vi "Main_UCRT_9.vi"() -> ()   [LabVIEW 2016]
doc: "Use this template to create an application that executes until you click the Stop button. Unlike the Single Loop Application VI that uses polling, this VI uses the Event Structure."
uses:
  <vilib>/vision/driver/NI_Vision_Acquisition_Software.lvlib
  <vilib>/vision/NI_Vision_Development_Module.lvlib
  Granule-2000AT/PC/Library.lvlib
  <vilib>/Utility/file.llb/Write To Spreadsheet File (string).vi
  <vilib>/Utility/file.llb/Read From Spreadsheet File (string).vi
  <vilib>/userdefined/High Color/IMAQdx.ctl
panel:
  in  "ND HEAT BUT":bool
  in  "ND HEAT LED":bool
  out "PT 4txt":string caption="Вакуум в камере\nPT2 (torr)"
  out "PT4 2":u16(ring)
  out "NL2":u16(ring)
  in  "V5014":dbl
  out "давление 2":bool
  out "давление 1":bool
  in  "V5012_SP_He_PC2":dbl
  out "Air":bool
  in  "ПЛАЗМАТРОН В ИСХОДНОЕ":bool
  in  "Продол назад":bool
  in  "V5011_SP_He_PC2":dbl
  in  "V5010_SP_C1":dbl
  out "PT 4":string caption="Вакуум в камере\nPT2 (torr)"
  in  "PT4":dbl
  in  "M_PLasmatron":dbl
  out "V барабаны 2":dbl
  in  "Tab Control 2":enum32{"X1", "X2", "Y"}(tab)
  out "X240":bool[](array[boolean])
  out "ОП1 Х1 5":string[](array[string])
  out "X200":bool[](array[boolean])
  out "ОП1 Х1 4":string[](array[string])
  out "X140":bool[](array[boolean])
  out "ОП1 Х1 3":string[](array[string])
  out "X100":bool[](array[boolean])
  out "ОП1 Х1 2":string[](array[string])
  out "X400":bool[](array[boolean])
  out "ОП1 Х1 8":string[](array[string])
  out "X340":bool[](array[boolean])
  out "ОП1 Х1 7":string[](array[string])
  out "X300":bool[](array[boolean])
  out "ОП1 Х1 6":string[](array[string])
  out "Y120":bool[](array[boolean])
  out "ОП1 Х1 10":string[](array[string])
  out "Y60":bool[](array[boolean])
  out "ОП1 Х1 9":string[](array[string])
  out "Air 4":bool
  in  "PT3 2":dbl
  in  "Запись отчета":bool
  out "V вращ. бараб 2":string caption="V заготовки"
  out "LONGITUDINAL SPEED":string
  out "PLASMATRON SPEED":string
  in  "mac3":bool
  in  "Ошибка 2":i16 format="%x"
  in  "Скорость пп 2":i16
  out "Полож заг сер":bool
  out "Полож заг нач":bool caption="НАЧАЛО"
  out "Полож заг кон":bool
  out "Полож плазм кон":bool caption="Конец"
  out "Полож плазм сер":bool caption="Пром."
  out "Полож плазм  нач":bool caption="Начало"
  in  "МАКСИМАЛЬНАЯ СКОРОСТЬ ПП К":bool
  in  "v4066_cкорость подачи плазматрона":dbl
  in  "v4065_cкорость подачи":dbl
  in  "V7045_I_ist":dbl
  in  "V7045_U_ist":dbl
  in  "Действующий ток на плазматроне":string caption="Ток А"
  out "V заготовки":string
  in  "D, заготовки":i16
  in  "Закончить автораспыление":bool
  in  "Автораспыление доплавить":bool
  in  "Автораспыление начать":bool
  in  "задание тока А":string caption="Задание, А"
  in  "ПОДАЧА ЗАГОТОВКИ":bool
  in  "stop 3":bool
  in  "stop 2":bool
  in  "SP_зазор":dbl
  in  "PV_зазор":dbl
  in  "max out":dbl
  in  "out":dbl
  out "Distance зазор":sgl format="%.2f"
  out "x/y":dbl
  out "x*y":dbl
  out "16bit integer":i16
  in  "Numeric":i16
  in  "Т6":dbl
  in  "Улавливатель закрыть":bool
  in  "Улавливатель открыть":bool
  in  "Ролик прижать":bool
  in  "Ролик отжать":bool
  in  "PE3":dbl
  in  "PE2":dbl
  in  "PE1":dbl
  in  "ЗАДАНИЕ ТОКА":i16
  in  "ГС - Закрыть":bool
  in  "ГС -Открыть":bool
  out "ГС - Плазматрон":string caption="Плазматрон"
  out "ГС - Камера":string caption="Камера"
  in  "Скорость пп":i16
  in  "V барабаны задание":dbl
  in  "Выход":bool
  in  "ГС ПТ":i16
  in  "ГС камера":i16
  in  "V барабаны":dbl
  in  "Т5":dbl
  in  "Т4":dbl
  in  "Т3":dbl
  in  "Т2":dbl
  in  "Т1":dbl
  in  "Ошибка":i16
  in  "PT3":dbl
  in  "PT2":dbl
  in  "PT1":dbl
  in  "y120":i32
  in  "y60":i32
  in  "x400":i32
  in  "x340":i32
  in  "x300":i32
  in  "x240":i32
  in  "x200":i32
  in  "x140":i32
  in  "x100":i32
  in  "Tab Control":enum32{"Вакуум", "Распыление", "Осциллограмма"}(tab)
  in  "откачка стоп 2":bool
  out "Распыление":bool
  out "Вакуум":bool
  out "Газ":bool
  out "VP4":u16(ring)
  out "SP Presure Ar PC2":string caption="SP C1 (kgf/cm^2)"
  in  "напустить аргон в ресивер":bool
  in  "mac6":bool
  out "SP Presure He PC2":string caption="SP C1 (kgf/cm^2)"
  in  "mac5":bool
  in  "напустить гелий в ресивер":bool
  out "SP Presure C1":string caption="SP C1 (kgf/cm^2)"
  in  "mac 4":bool
  in  "напустить газ в камеру":bool
  out "PD2":u16(ring)
  out "VP2":u16(ring)
  in  "forvacuum":bool
  in  "forvakuum led":bool
  in  "Slide":dbl(slide) scale=0.0..99.0
  in  "откачка стоп":bool
  in  "откачка стоп индик":bool
  out "EV1":u16(ring)
  out "EV2":u16(ring)
  out "EV3.3":u16(ring)
  out "EV3.2":u16(ring)
  out "PE2":u16(ring)
  out "PE2":string caption="Вакуум в камере\nPT2 (torr)"
  out "CO1":u16(ring)
  out "CO2":u16(ring)
  out "EV3.1":u16(ring)
  out "CO3":u16(ring)
  out "P1":u16(ring)
  out "PE1":u16(ring)
  out "PE1":string caption="Вакуум в камере\nPT2 (torr)"
  out "PE3":u16(ring)
  out "PE3":string caption="Вакуум в камере\nPT2 (torr)"
  out "VP1":u16(ring)
  out "PT3":u16(ring)
  out "PT2":u16(ring)
  out "PT 2":string caption="Вакуум в камере\nPT2 (torr)"
  out "VP3":u16(ring)
  out "VP5":u16(ring)
  out "PD1":u16(ring)
  out "PT1":u16(ring)
  out "PT 1":string caption="Вакуум в камере\nPT2 (torr)"
  out "NZ1":u16(ring)
  out "NR1":u16(ring)
  out "NL1":u16(ring)
  in  "откачать рабочий вакуум":bool
  in  "mac 2":bool
  out "PT 3":string caption="Вакуум в камере\nPT2 (torr)"
  out "ИНдикатор положения полки":string
  in  "ЗУ-вверх":bool
  in  "Пауза допыления":string caption="Пауза допыления (sec)"
  out "C212":bool
  out "УГ_закрыт":bool caption="Отжат"
  out "УГ_открыт":bool caption="Прижат"
  out "ролик_отжат":bool caption="Вверху"
  out "ролик_прижат":bool caption="Внизу"
  out "max Speed":string caption="Максимальная \nСкорость (r/min)"
  out "ТЕМП КАМЕРА":string caption="T газ (C°)"
  in  "Скорость ПП 2":string caption="Скорость плазматрона\n(mm/min)"
  in  "Скорость ПП":string caption="Скорость толкателя (mm/min)"
  out "ТЕМП РОЛИК":string caption="T ролик (C°)"
  out "ПОДШ. 2.2":string caption="T4 (C°)"
  out "ПОДШ. 2.1":string caption="T3 (C°)"
  out "ПОДШ. 1.2":string caption="T2 (C°)"
  out "ПОДШ. 1.1":string caption="T1 (C°)"
  out "P плазматрон (bar)":string
  out "P камера (bar)":string
  out "I_ist":string caption="Ток (A)"
  out "U_ist":string caption="Напряжение (V)"
  in  "Tab Control 3":enum32{"Настройки видео", "Регулятор"}(tab)
  in  "Media Stop Button":bool
  in  "Play Button":bool
  in  "Камера":T1
  in  "Область измерения":T2 {"Rotation" format="%.2f"; "Left" scale=0.0..1024.0; "Right" scale=0.0..1280.0}
  in  "Параметры измерения":T3={"Contrast"=40, "Filter width"=4, "Steepness"=2, "Subsampling Ratio"=5, "Show Search Area"=FALSE, "Show Search Lines"=FALSE, "Show Edges Found"=FALSE, "Show Result"=TRUE}
  in  "Рабочий цвет":u32(colorbox)
  in  "Калибровка":u32(colorbox)
  in  "Задержка":u32
  in  "Уровень бинаризации":T4={"Нижний предел"=128.0, "Верхний предел"=255.0} {"Верхний предел" format="%.2f"; "Нижний предел" format="%.2f"}
  in  "Фильтр":i32(ring)=1 items=["Red", "Green", "Blue", "Hue", "Saturation", "Luminance", "Value", "Intensity"]
  out "Индикатор камеры":bool
  in  "Blank Button":bool
  out "Индикатор камеры 2":bool
  in  "Сохранить настройки":bool
  in  "автоматическое включение регулятора":bool caption="Автоматическое включение регулятора"
  out "Индикатор автозапуска регулятора":bool
  out "Запись":bool
  out "Максимальная подача (мм/мин)2":string caption="Max скорость\n(mm/min)"
  out "Boolean":bool
  in  "Регулятор":bool
  out "текущая скорость\n(mm/min)":string
  out "текущее значение\nзазора (mm)":string
  out "Задание \nзазора (mm)":string
  in  "взять зазор":bool caption="Регулятор"
  out "Марка сплава":string
  out "Порядковый номер":string caption="Номер цикла (un)"
  in  "Положение толкателя (mm)":dbl(slide) scale=0.0..100.0
  out "Диаметр заг.":string caption="Диаметр (mm)"
  out "V задания":string caption="Скорость вращения (r/min)"
  out "V вращ. бараб":string caption="Частота вращения (r/min)"
  in  "Продол впер":bool
  out "индикация видео":T5(plugin-control)
  in  "ПЛАЗМАТРОН В ИСХОДНОЕ 2":bool
  out "Частота вращения":dbl(graph)
  out "Значение зазора":dbl(graph)
  out "Скорость толкателя":dbl(graph)
  out "Ток":dbl(graph)
  out "Напряжение":dbl(graph)
  out "voto plasmatron":string caption="моточасы работы\nплазматрона"
  out "текущее время":string
  in  "Arhive":bool
  # "Ролик"
  # "Улавливатель ОГ"
  # "PLASMATRON"
  # "Обработка"
  # "БАРАБАНЫ"
  # "РАСПЫЛЕНИЕ ЗАГОТОВКИ"
  # "Температура"
  # "3A3.1 X100-X137"
  # "3A3.2 X140-177"
  # "3A4 X200-X237"
  # "3A5.1 X240-X277"
  # "3A5.2 X300-X337"
  # "3A6 X340-X377"
  # "3A8 X400-X437"
  # "2A8 Y60-Y117"
  # "3A7 Y120-Y157"
  # "Положение толкателя"
  # "Положение плазматрона"
  # "Газовая система"
  # "VF1"
  # "Ar,He"
  # "PC1"
  # "PC2"
  # "Толкатель"
  # "Прижим крышки"
  # "Прижимной ролик"
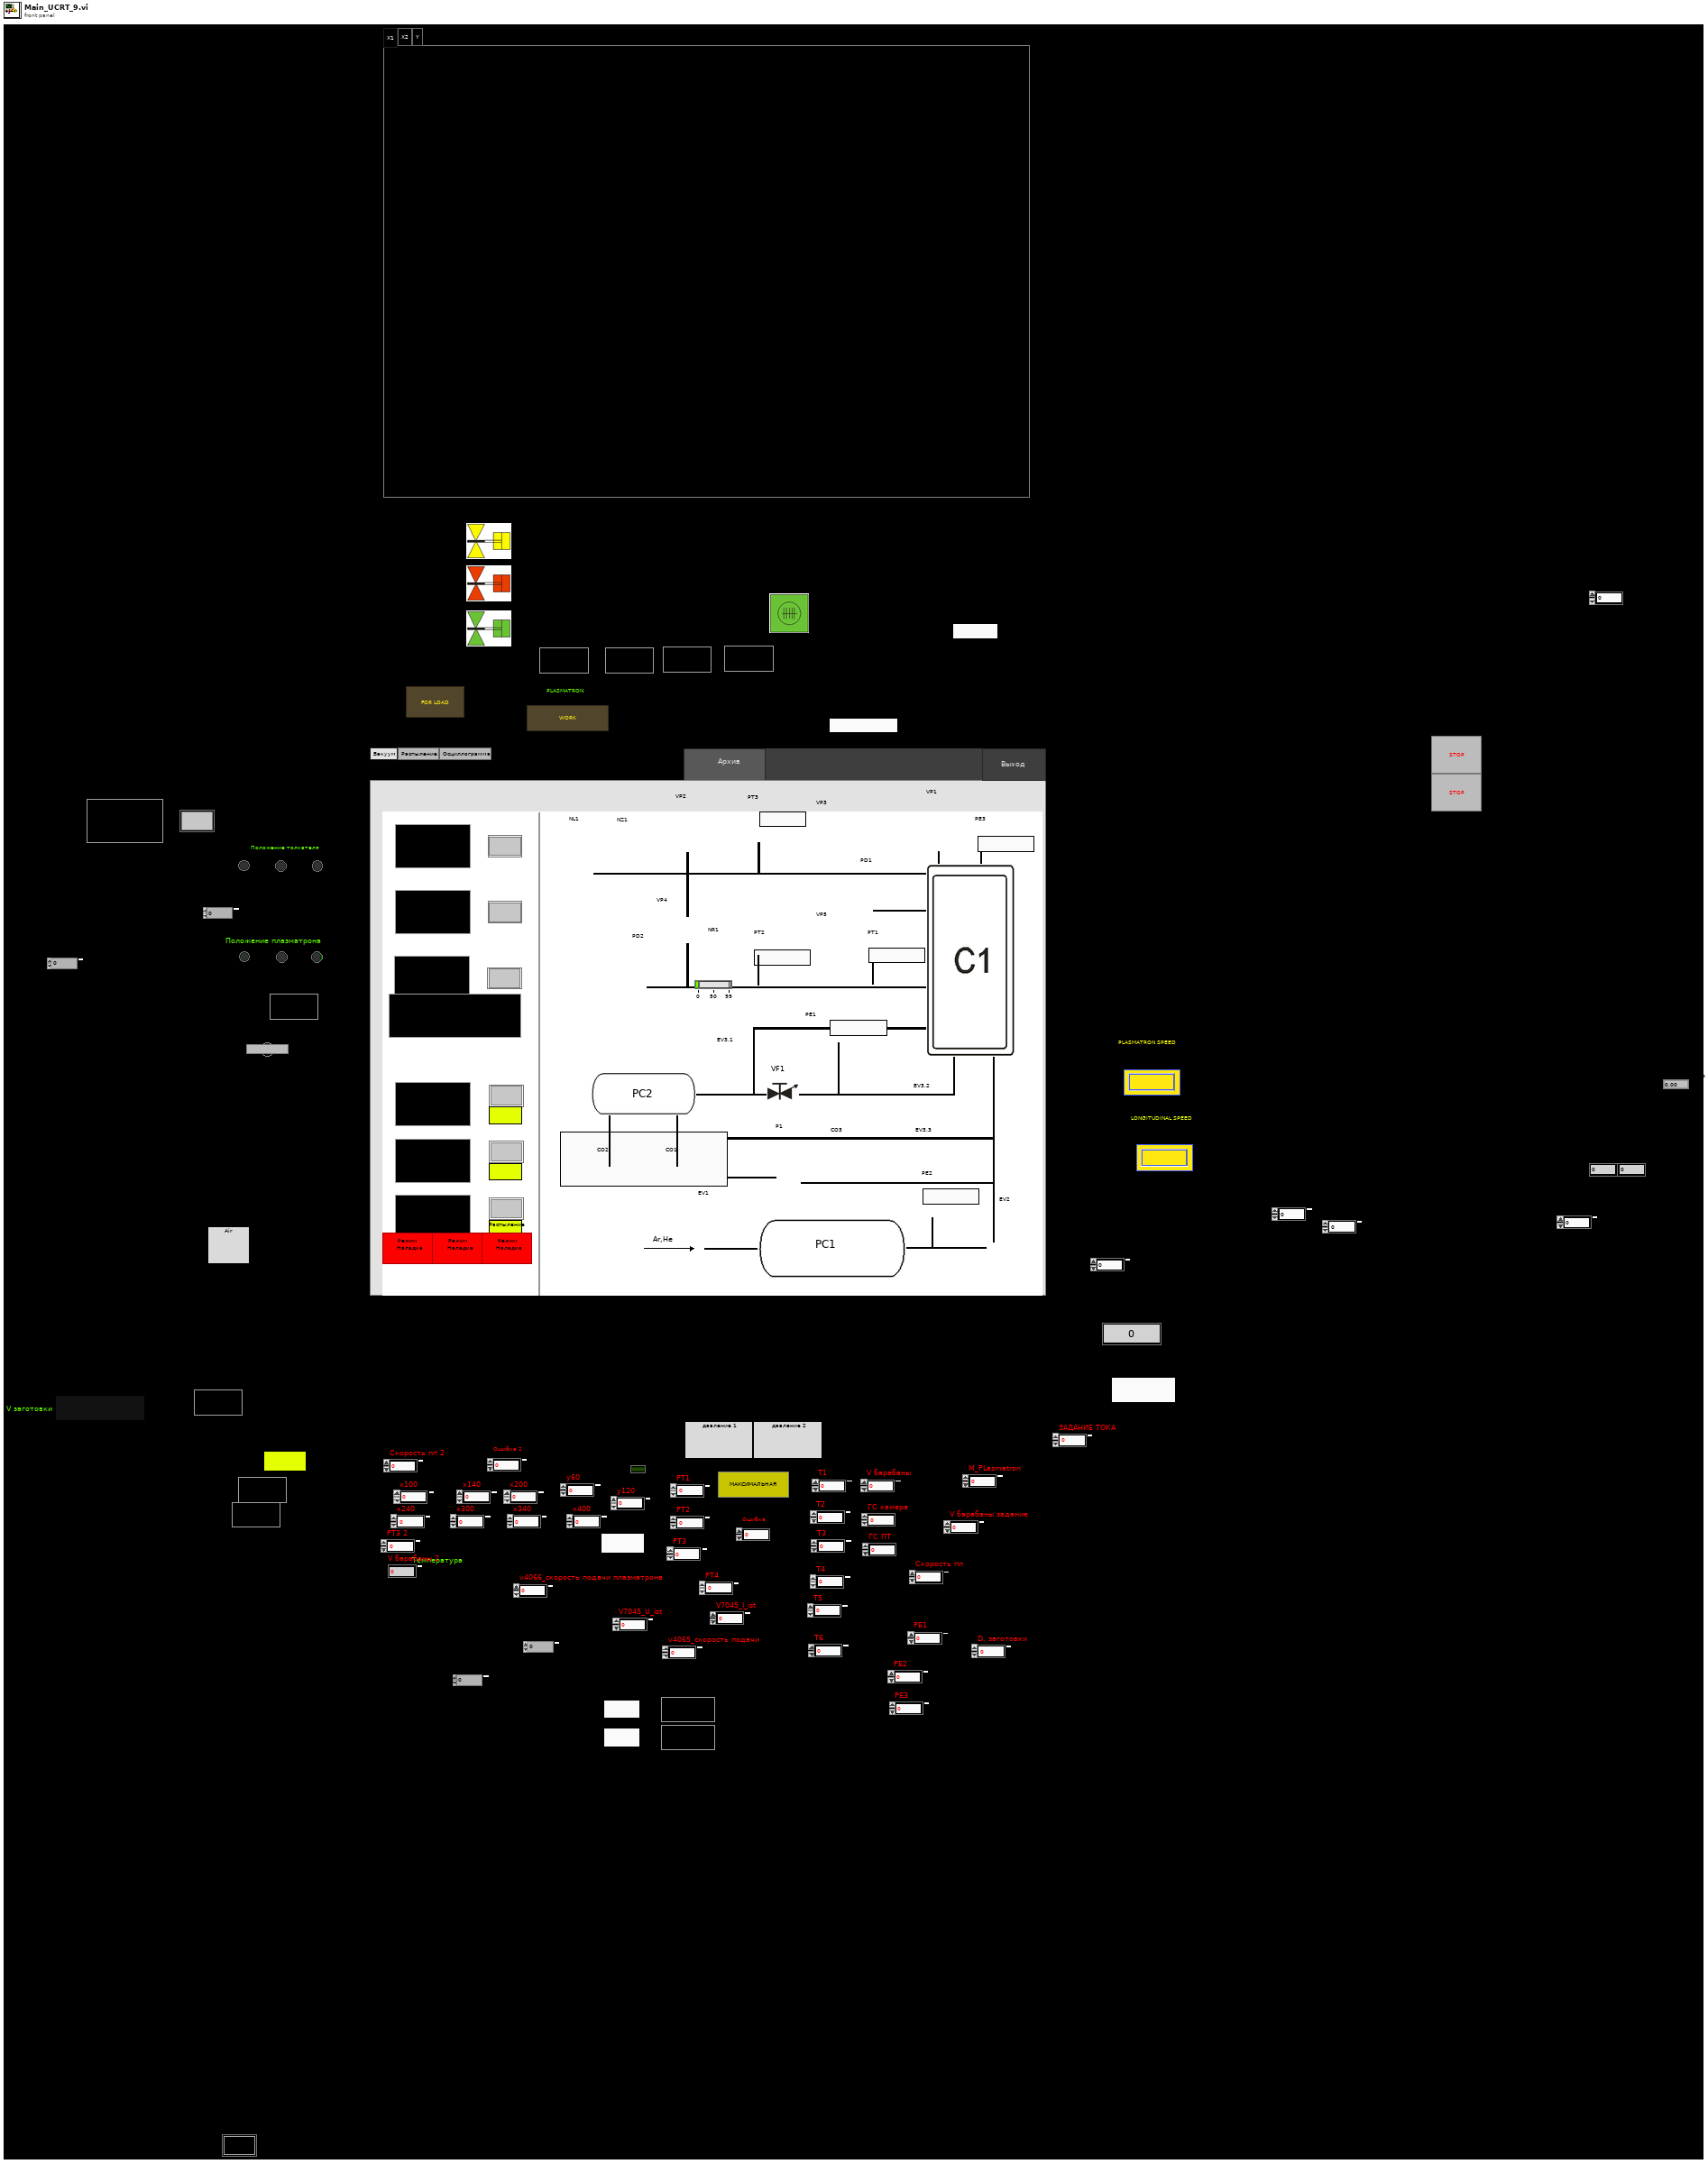
[diagram p1: front panel]
types:
  T1 = typedef "IMAQdx.ctl" = refnum<k21>
  T2 = typedef "IMAQ Rectangle" = cluster{"Left":i32, "Top":i32, "Right":i32, "Bottom":i32, "Rotation":dbl}
  T3 = cluster{"Contrast":i32, "Filter width":i32, "Steepness":i32, "Subsampling Ratio":u32, "Show Search Area":bool, "Show Search Lines":bool, "Show Edges Found":bool, "Show Result":bool}
  T4 = cluster{"Нижний предел":sgl, "Верхний предел":sgl}
  T5 = typedef "IMAQ Image.ctl" = refnum<image>
  T6 = enum16{"open", "replace", "create", "open or create", "replace or create", "replace or create with confirmation"}
  T7 = enum8{"Enabled", "Disabled", "Disabled and Grayed Out"}
  T8 = cluster{i32, i32, i32, u32, "Boolean":bool, "Boolean":bool, "Boolean":bool, "Boolean":bool}
  T9 = typedef "Image Type" = u32
  T10 = typedef "Library.lvlib/IMAQdx.ctl" = refnum<k21>
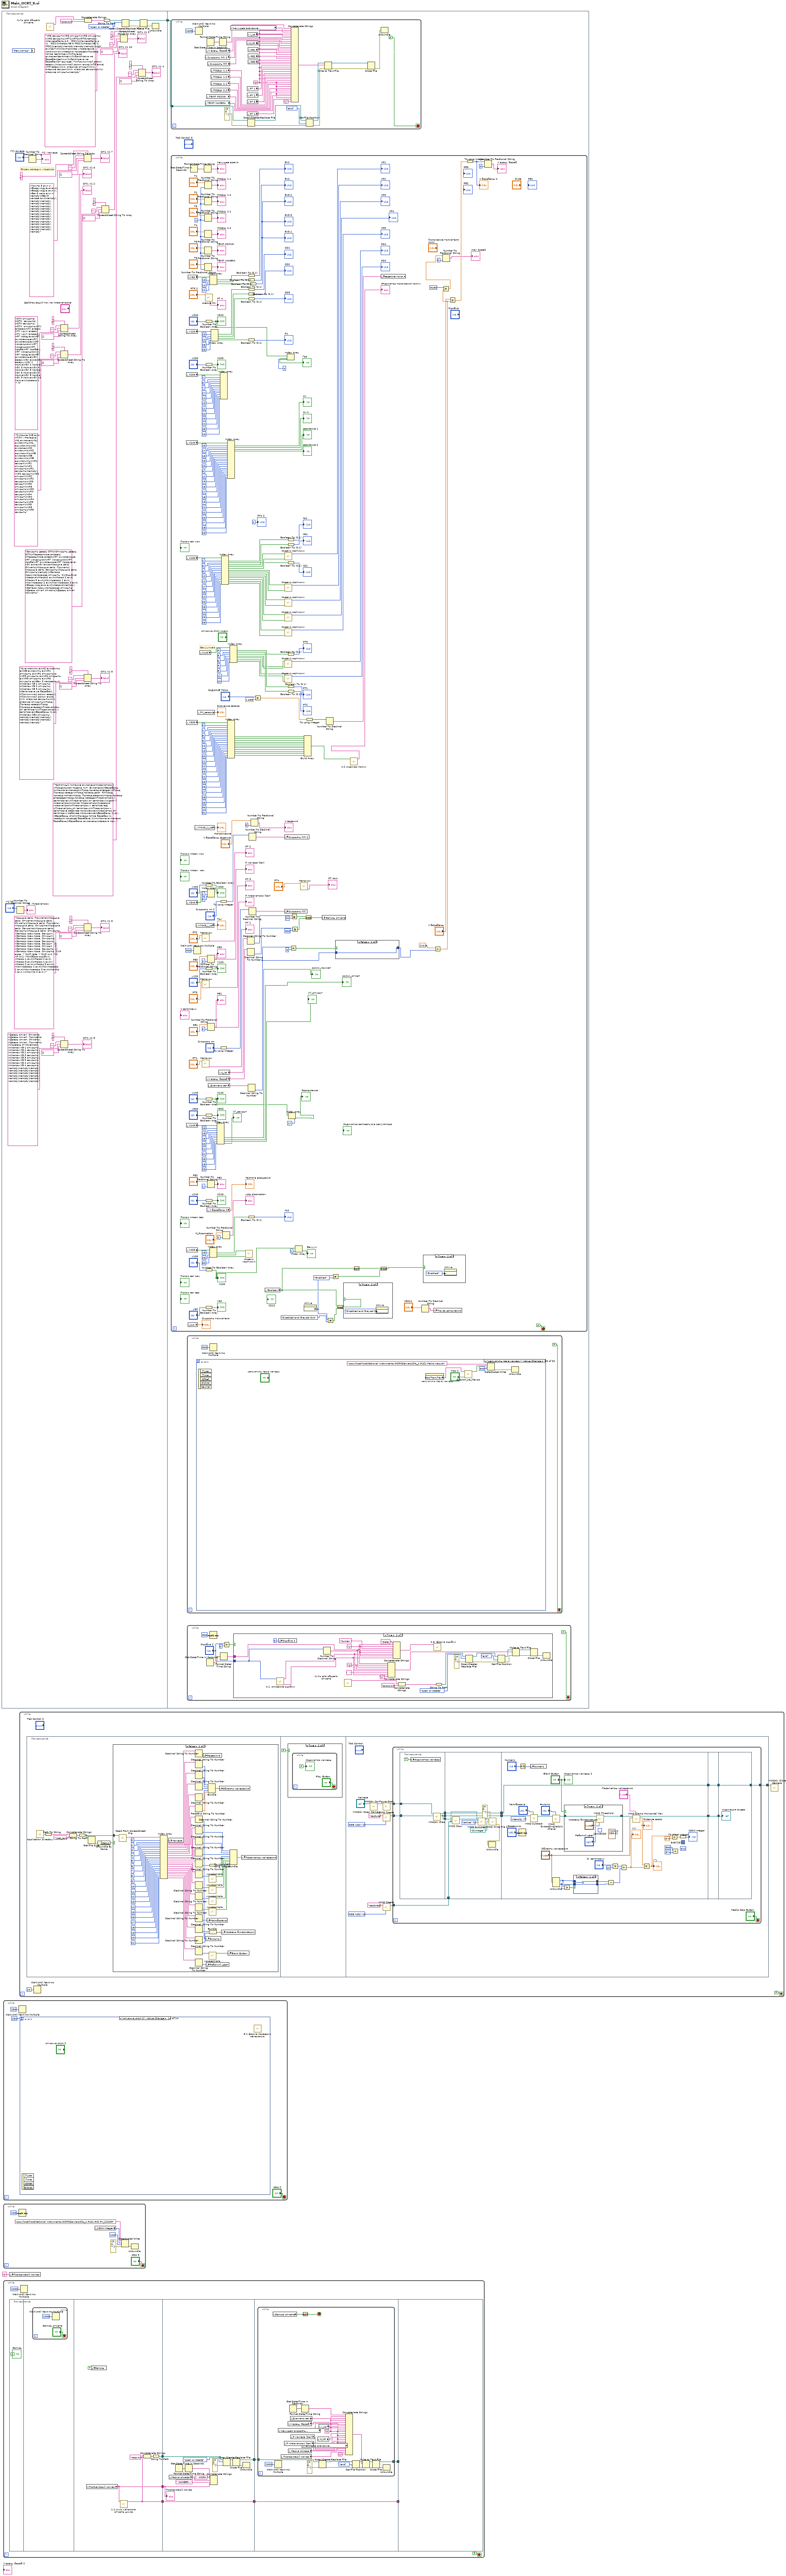
[diagram p0: block diagram]
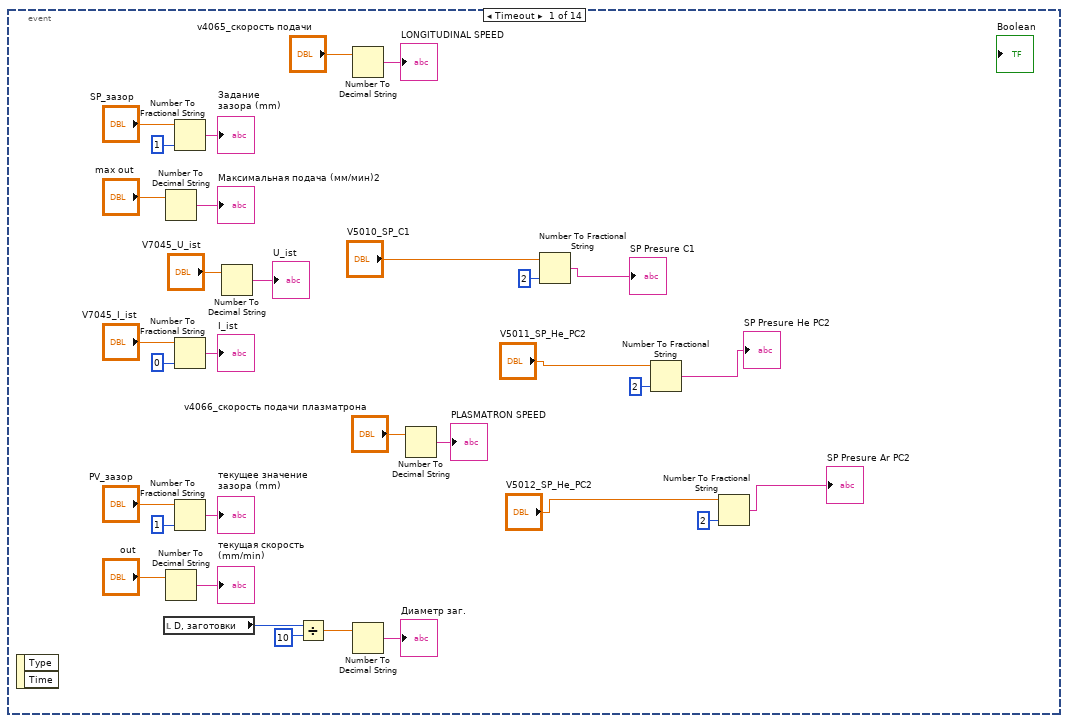
[diagram p6: hidden frame]
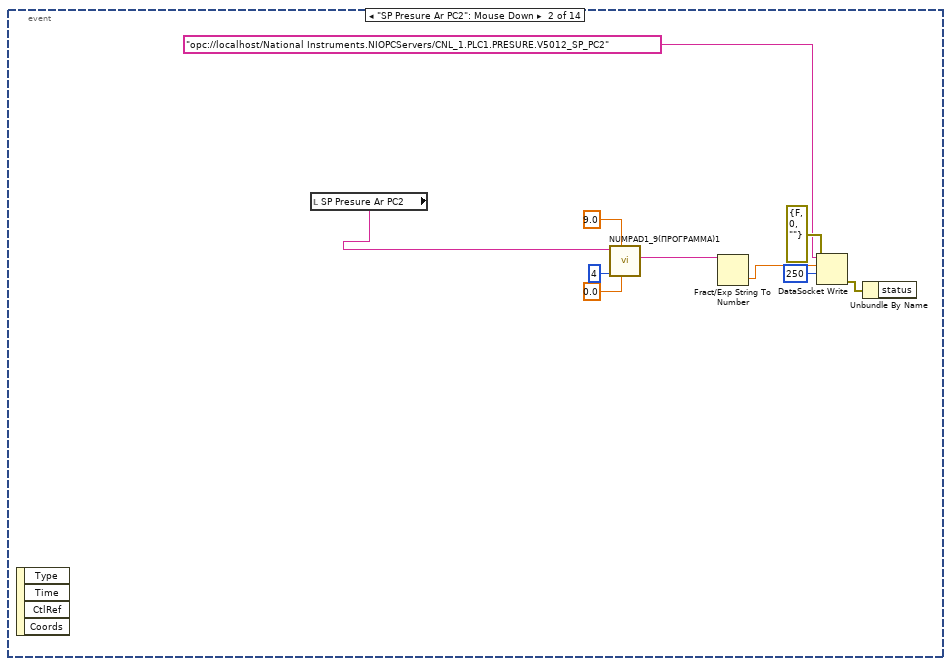
[diagram p7: hidden frame]
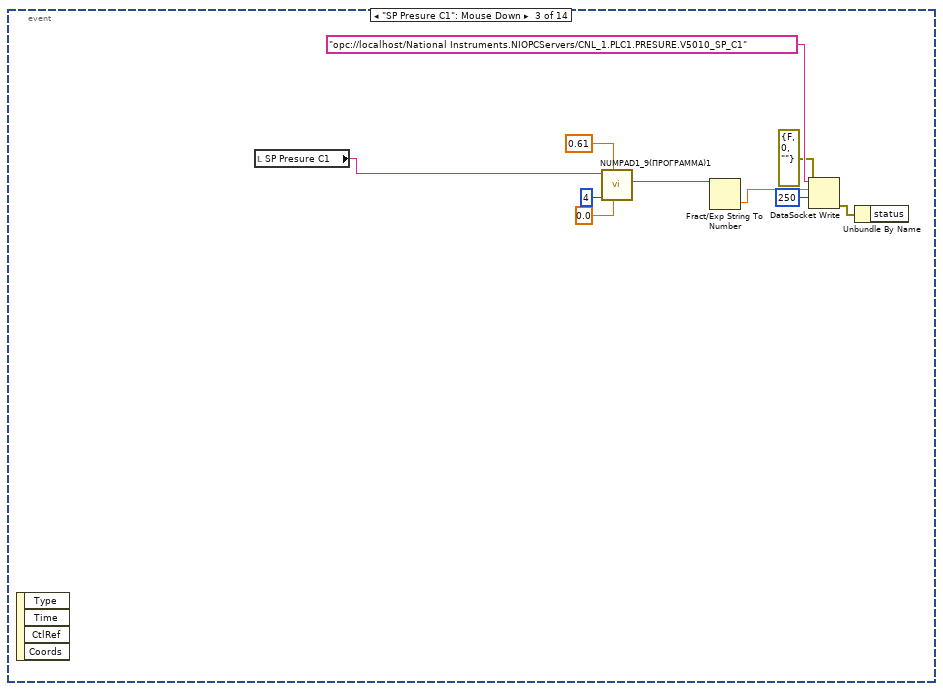
[diagram p8: hidden frame]
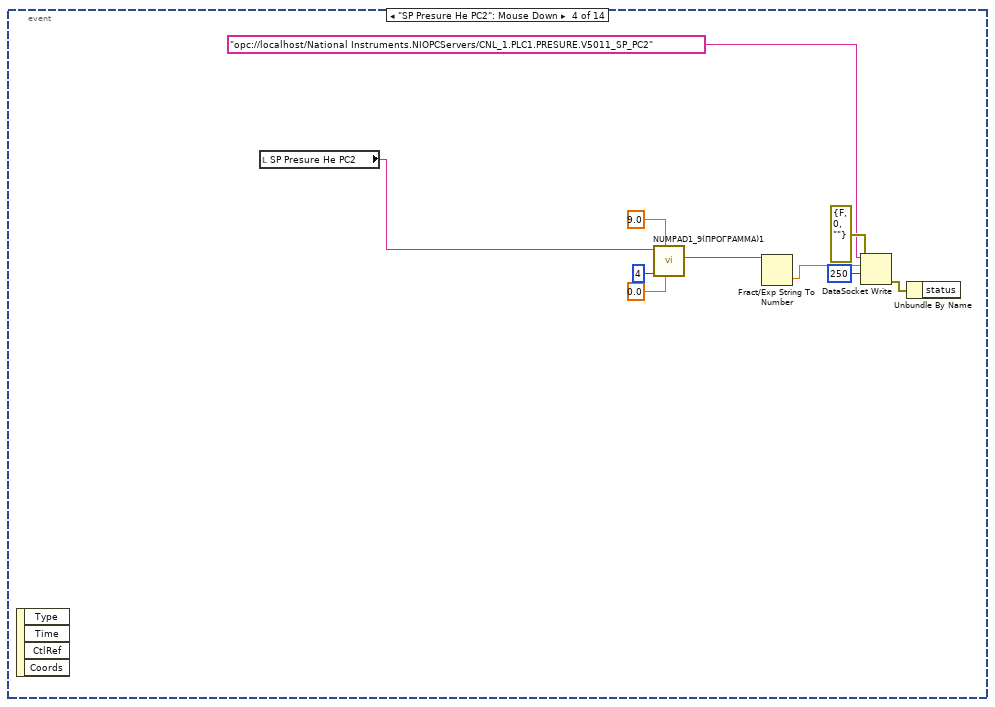
[diagram p9: hidden frame]
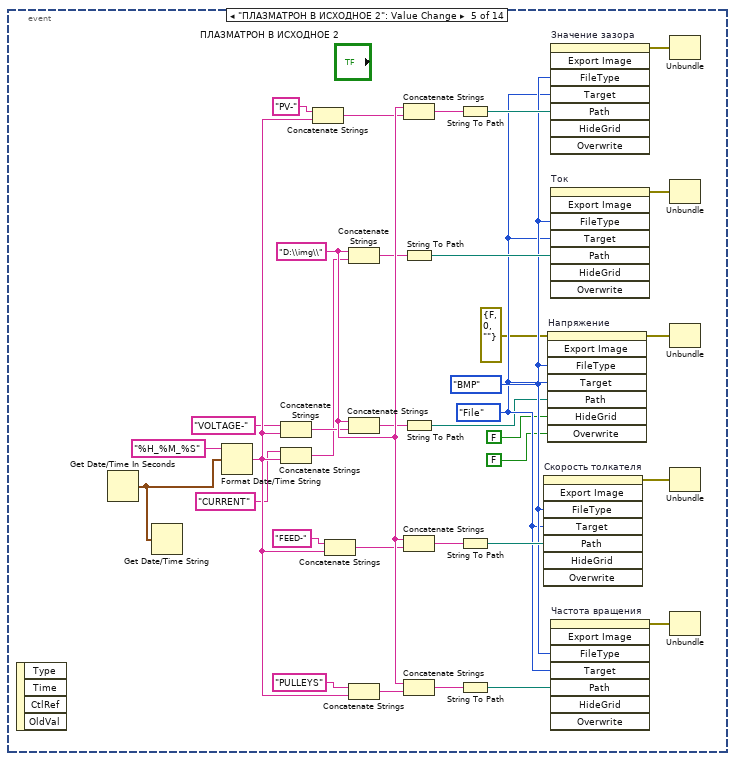
[diagram p10: hidden frame]
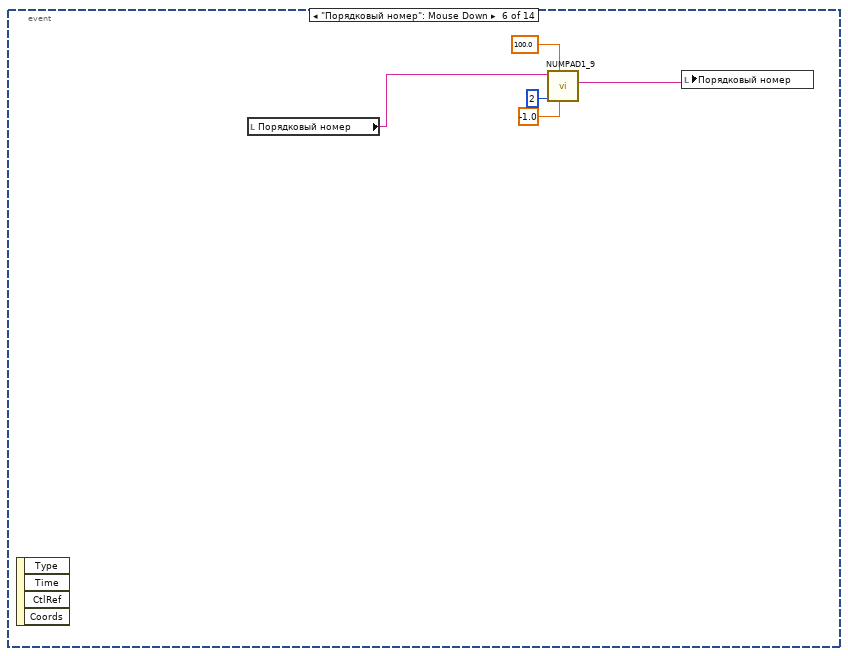
[diagram p11: hidden frame]
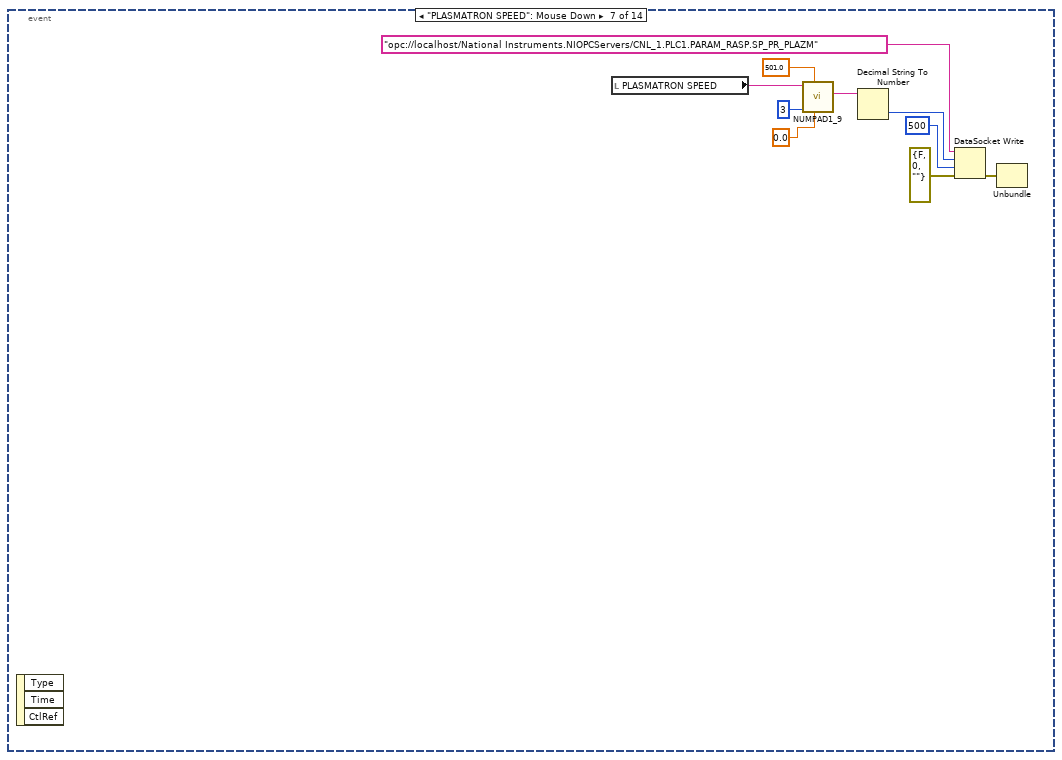
[diagram p12: hidden frame]
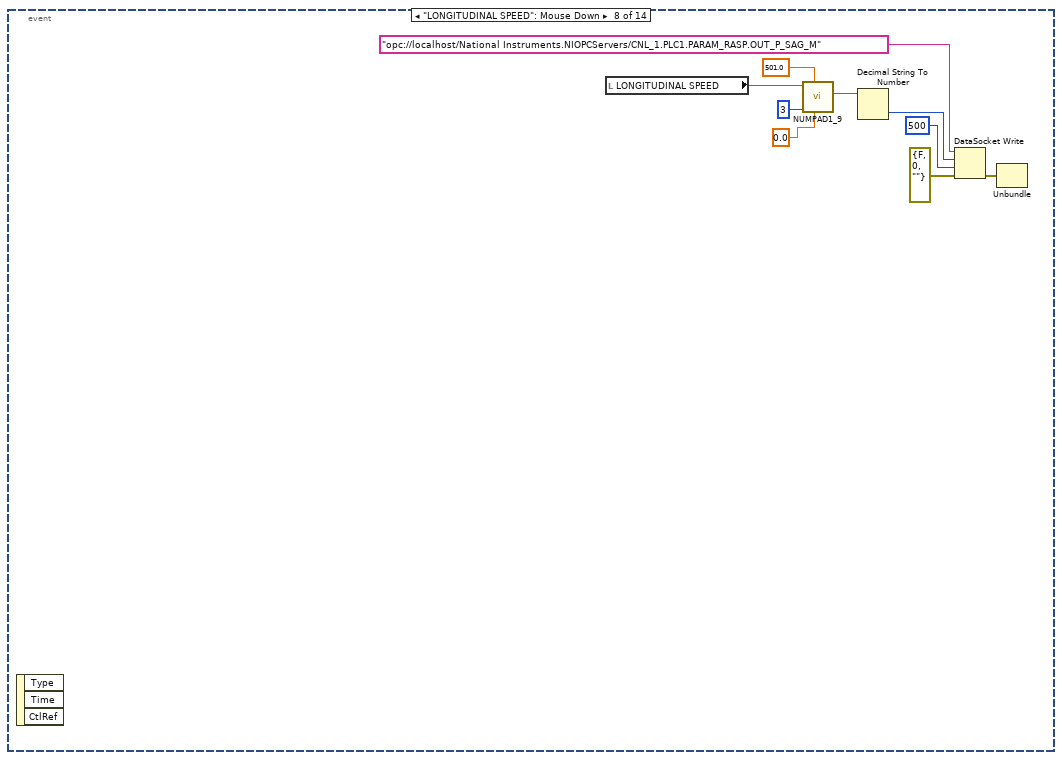
[diagram p13: hidden frame]
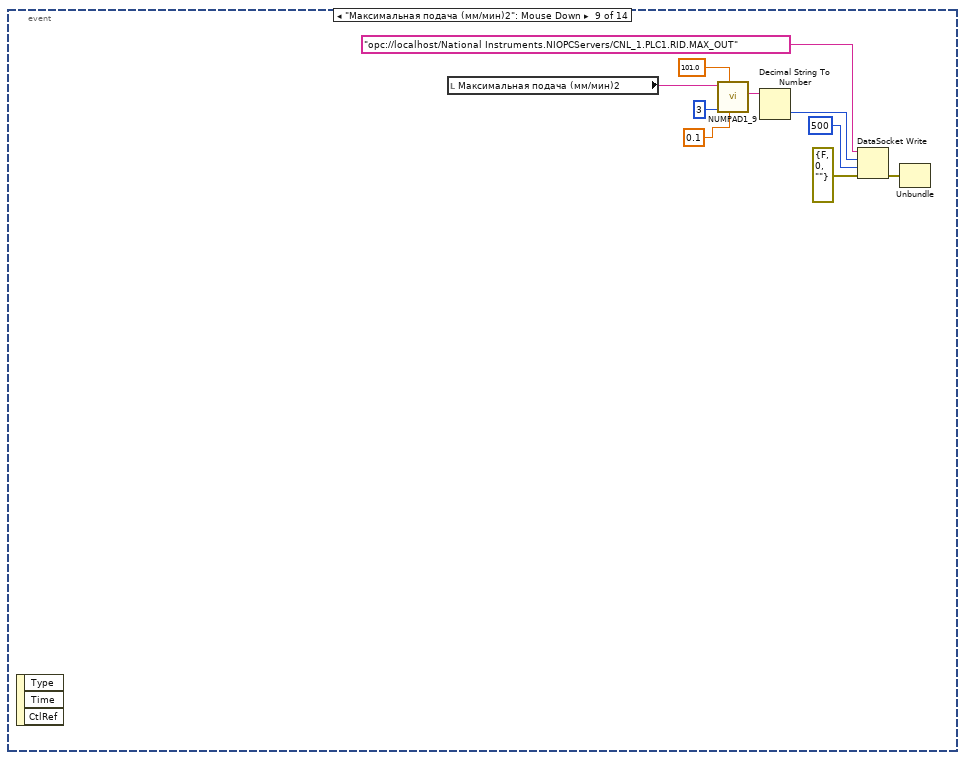
[diagram p14: hidden frame]
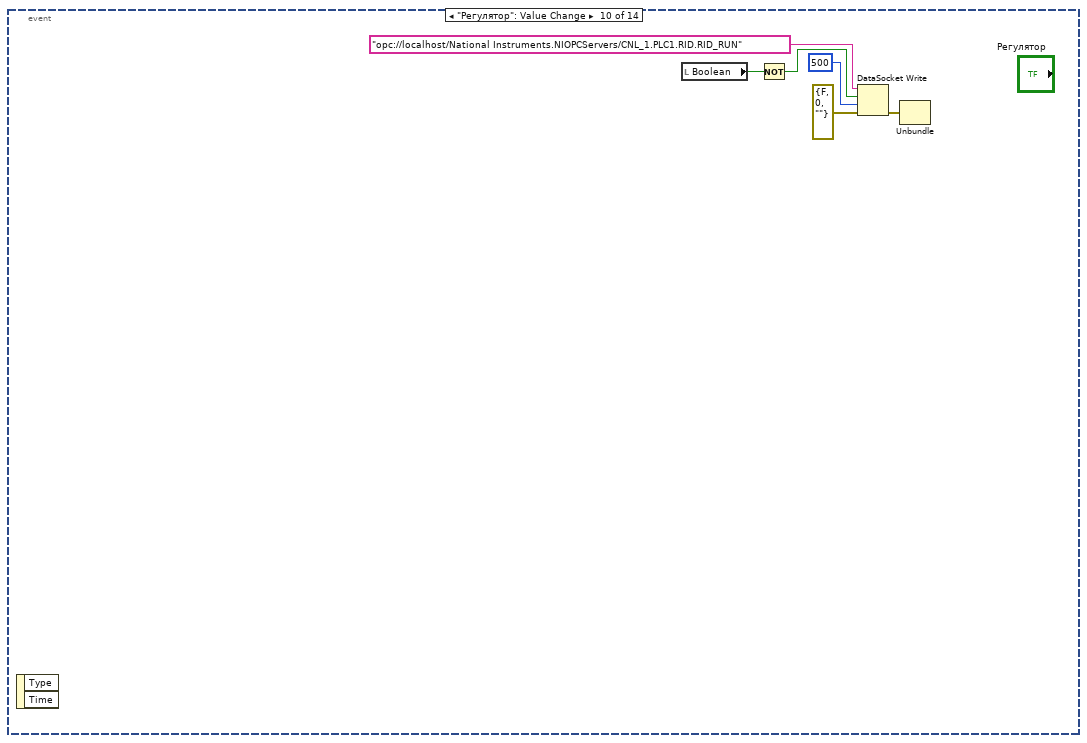
[diagram p15: hidden frame]
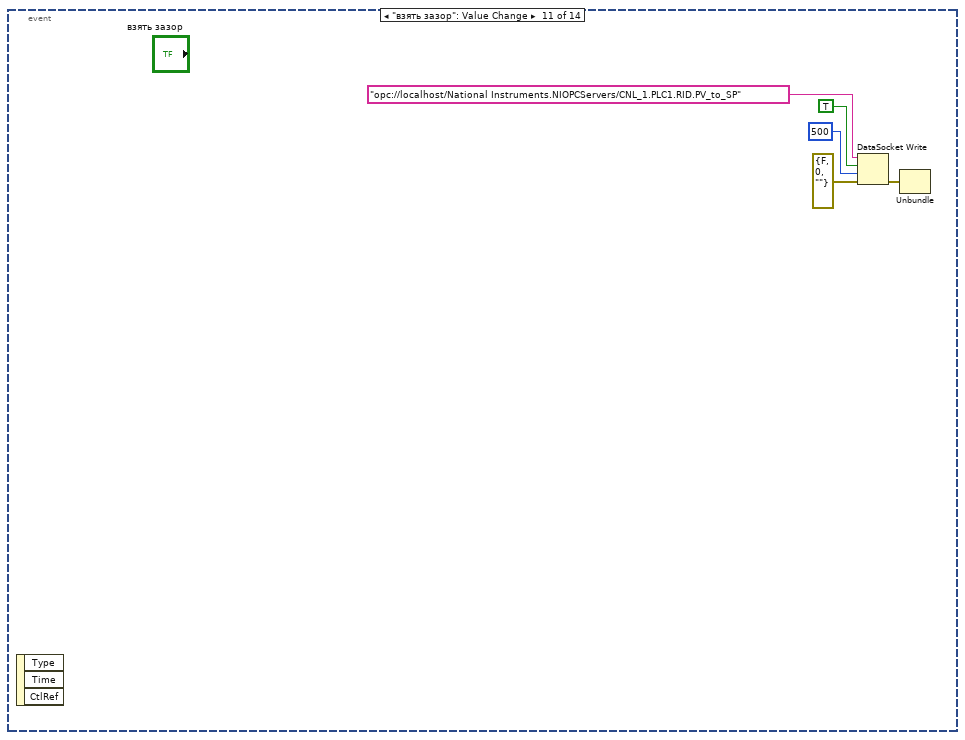
[diagram p16: hidden frame]
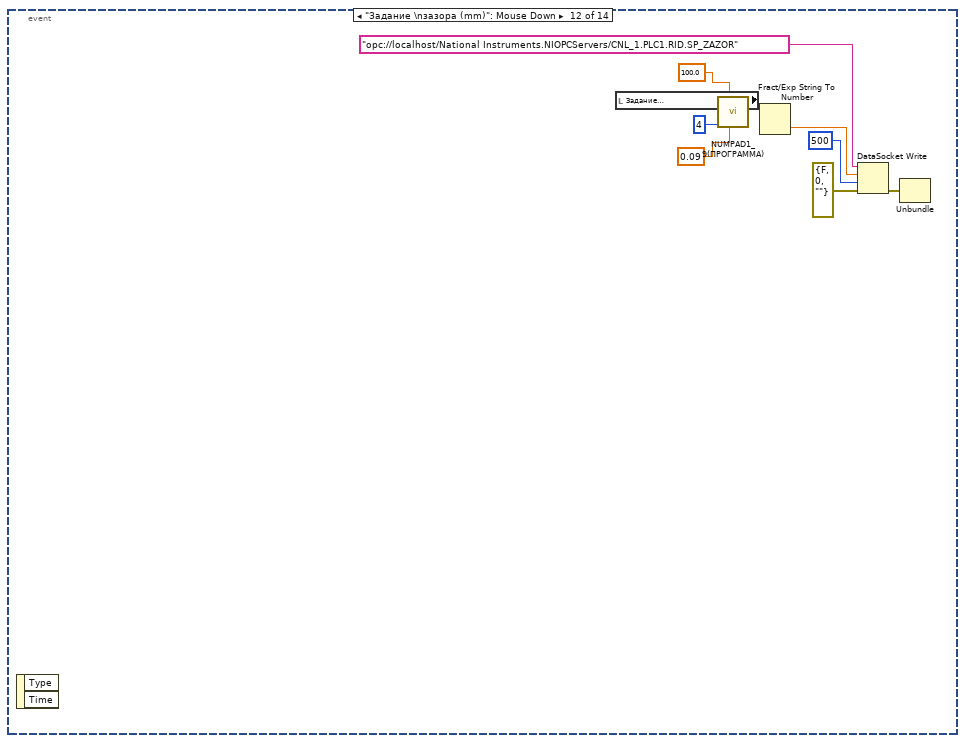
[diagram p17: hidden frame]
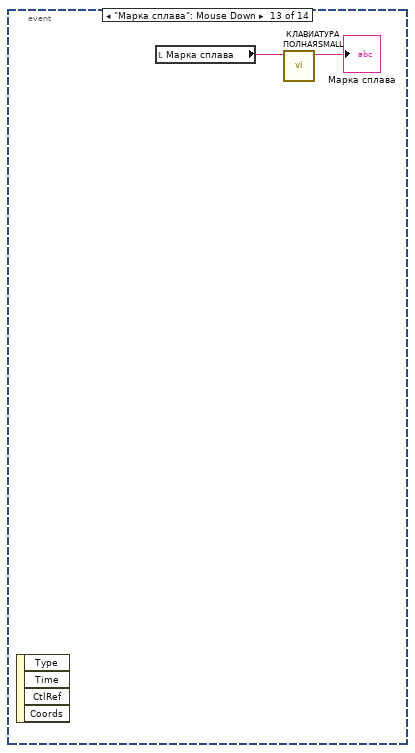
[diagram p18: hidden frame]
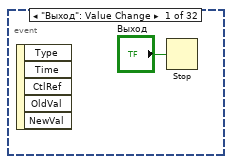
[diagram p20: hidden frame]
diagram:
  n1 = flat-sequence {
    tunnel: [w4] -> w1
    tunnel: w1 -> [w62]
    frame #0 {
      # "Экран наладки - подписи"
      n2 = local write "Tab Control 3"(enum32{"Настройки видео", "Регулятор"}."Регулятор" ("Tab Control 3")) -> ()
      n3 = Number To Decimal String(number="ГС ПТ") -> (decimal integer string=→"ГС - Плазматрон":string)  [unwired: 1 in]
      n4 = Number To Decimal String(number="ГС камера") -> (decimal integer string=→"ГС - Камера":string)  [unwired: 1 in]
      n5 = call "путь для общего отчета.vi"() -> ("path_out 2"=w10:string)  [unwired: 11 in]
      n6 = Spreadsheet String To Array(delimiter (Tab)="\n", format string="", spreadsheet string="ОТК открыта\nОТК  закрыта\nОТК закрыть\nОТК  открыть\nПУ вправо\nПУ влево\nПУ крут влево\nПУ крут вправо\nРГ продувка\nРГ окисленные\nРГ окисленныек\nРГ кондиционк\nРГ кондицион\nРГ проба\nРГ пробак\nРГ кондиционкк\nРГ продувка\nРГ окисленные\nЗУ вверх\nЗУ вниз\nЗУ вверху\nЗУ 1 полка\nЗУ 2 полка\nЗУ 3 полка\nЗУ 4 полка\nЗУ 5 полка\nЗУ 6 полка\nЗУ 7 полка\nЗУ 8 полка\nЗУ 9 полка\nЗУ 10 полка\nУровень 1 < N", array type (2D Dbl)=string[] [] ("ОП1 Х1")) -> (array=→"ОП1 Х1 6":string[])
      n7 = Spreadsheet String To Array(delimiter (Tab)="\n", format string="", spreadsheet string="Питание 24В вкл\nПЛК / Наладка\nNL включен\nNL включить\nNL выключить\nNZ включен\nNZ включить\nNZ выключить\nNB включен\nNB включить\nNB выключить\nVP1 закрыт\nVP1 открыт\nVP1 открыть\nVP1 закрыть\nempty\nVP2 закрыт\nVP2 открыт\nVP2 открыть\nVP2 закрыть\nVP3 закрыт\nVP3 открыт\nVP3 открыть\nVP3 закрыть\nVP4 закрыт\nVP4 открыт\nVP4 открыть\nVP4 закрыть\nVP5 закрыт\nVP5 открыт\nVP5 открыть\nVP5 закрыть", array type (2D Dbl)=string[] [] ("ОП1 Х1")) -> (array=→"ОП1 Х1 2":string[])
      n8 = Spreadsheet String To Array(delimiter (Tab)="\n", format string="", spreadsheet string="Дверь откат. Отжата\nДверь откат. Прижата\nДверь откат. Отжать\nДверь откат. Прижать\nУровень 3<N\nempty\nКлапан КЭ 1 открыть\nКлапан КЭ 1 закрыть\nКлапан КЭ 2 открыть\nКлапан КЭ 3 закрыть\nКлапан КЭ 3 открыть\nКлапан КЭ 3 закрыть\nКлапан КЭ 4 открыть\nКлапан КЭ 4 закрыть\nempty\nempty\nempty\nempty\nempty\nempty\nempty\nempty\nempty\nempty\nempty\nempty\nempty\nempty\nempty\nempty\nempty\nempty", array type (2D Dbl)=string[] [] ("ОП1 Х1")) -> (array=→"ОП1 Х1 8":string[])
      n9 = Spreadsheet String To Array(delimiter (Tab)="\n", format string="", spreadsheet string="Компр 3 вкл к\nВоздуходувка вкл\nВоздуходув вкл к\nБак3 нагр вкл к\nempty\nБак3 нагрев вкл\nempty\nempty\nempty\nempty\nempty\nempty\nempty\nempty\nempty\nempty\nempty\nempty\nempty\nempty\nempty\nempty\nempty\nempty\nempty\nempty\nempty\nempty\nempty\nempty\nempty\nempty", array type (2D Dbl)=string[] [] ("ОП1 Х1")) -> (array=→"ОП1 Х1 7":string[])
      n10 = Spreadsheet String To Array(delimiter (Tab)="\n", format string="", spreadsheet string="NL включить в\nNZ включить в\nNB включить в\nVP1 открыть в\nVP2 открыть в\nVP3 открыть в\nVP4 открыть в\nVP5 открыть в\nVP6 открыть в\nБак 3 нагрев вкл\nКлапан КЭ 1 открыть\nКлапан КЭ 2 открыть\nКлапан КЭ 3 открыть\nЗаготовка на барабан\nПрижимной ролик вверх\nПрижимной ролик вниз\nУл. огарков закрыть\nУл. огарков открыть\nПрод. Привод назад\nПрод. Привод вперед\nПлазматрон от заготовки\nПлазматрон к заготовке\nБарабаны пуск\nКлапан КЭ4 открыть\nempty\nempty\nempty\nempty\nempty\nempty\nempty\nempty", array type (2D Dbl)=string[] [] ("ОП1 Х1")) -> (array=→"ОП1 Х1 9":string[])
      n11 = Spreadsheet String To Array(delimiter (Tab)="\n", format string="", spreadsheet string="Крышка загр. Прижата\nКрышка загр. Отжата\nКрышка загр. Отжать\nКрышка загр. Прижать\nКрышка загр. Открыта\nКрышка загр. Закрыта\nКрышка загр. Закрыть\nКрышка загр. Открыть\nЗатвор гран.пров. Закрыт\nЗатвор гран.пров. Открыт\nЗатвор гран.пров. Открыть\nЗатвор гран.пров. Закрыть\nЗатвор гран.пров. Закрыт   2\nЗатвор гран.пров. Открыт   2\nЗатвор гран.пров. Закрыть  2\nЗатвор гран.пров. Открыть  2\nP возд. < N\nP газа < N\nP нк1 <N\nP нк2 <N\nСброс ошибки\nНасос 1 вкл\nНасос 2 вкл\nНасос 3 вкл\nНасос 1 вклк\nНасос 2 вклк\nНасос 3 вклк\nКомпрессор 1 вкл\nКомпрессор 2 вкл\nКомпрессор 3 вкл\nКомпр 1 вкл к\nКомпр 2 вкл к", array type (2D Dbl)=string[] [] ("ОП1 Х1")) -> (array=→"ОП1 Х1 5":string[])
      n12 = Concatenate Strings(w10, "proc.txt") -> (w12:string)
      n13 = Spreadsheet String To Array(delimiter (Tab)="\n", format string="", spreadsheet string="Закрыть дверь ОТК\nОткрыть дверь ОТК\nПересыпное вправо\nПересыпное влево\nРГ окисленные\nРГ кондицион\nРГ кондицион\nРГ проба\nРГ окисленные\nРГ продувка\nЗУ вниз\nЗУ вниз\nКрышка загр. Отжать\nКрышка загр. Прижать\nКрышка загр. Закрыть\nКрышка загр. Открыть\nempty\nЗатвор гранулопровода открыть  2\nОшибка\nАвария\nНасос1 вкл\nНасос 2 вкл\nНасос 3 вкл\nКомпрессор 1 вкл\nКомпрессор 2 вкл\nКомпрессор 3 вкл\nВоздуходувка вкл\nАвария\nempty\nЗатвор гранулопровода открыть\nДверь откат отжать\nДверь откат прижать", array type (2D Dbl)=string[] [] ("ОП1 Х1")) -> (array=→"ОП1 Х1 10":string[])
      n14 = String To Path(string=w12) -> (path=w8:path)
      n15 = Spreadsheet String To Array(delimiter (Tab)="\n", format string="", spreadsheet string="VP6 закрыт\nVP6 открыт\nVP6 открыть\nVP6 закрыть\nPT1\nPT2\nPT3\nempty\nКамераЗагруз 0   (PD1)\nКамераЗагруз -1   (PD1)\nНасос NB 0 (PD2)\nНасос NB -1 (PD2)\nempty\nempty\nempty\nempty\nИст вкл(ДУГА)\nКонтроллер управление источником\nАвария привода\nПривод готов (заготовки)\nПривод включен(заготовки)\nЗаготовка на барабан(датчик)\nЗаготовка на барабан(от выхода Y)\nПрижимной ролик вверху\nприжимной ролик внизу\nПР вниз\nПР вверх\nУл. огарков открыт\nУл. огарков закрыт\nУл. огарков закрыть\nУл. огарков открыть\nempty", array type (2D Dbl)=string[] [] ("ОП1 Х1")) -> (array=→"ОП1 Х1 3":string[])
      n16 = Open/Create/Replace File(file path (use dialog)=w8, operation (0:open)=T6."open or create") -> (refnum out=w5:refnum<file>, error out=w6:errorcluster)  [unwired: 4 in, 1 out]
      n17 = Spreadsheet String To Array(delimiter (Tab)="\n", format string="", spreadsheet string="Частотный питание включено(плазматрон)\nПродольная подача пит. Включено\nБарабаны питание включено\nПрод.привод впередк\nПрод. Привод назадк\nПрод привод дост. F\nПрод.привод готов\nпрод. Привод авария\nпрод.привод впередд\nпрод.привод назадд\nПлазматрон к заготовкек\nПлазматрон от заготовки\nдост f   плазматрон\nготов (плазматрон)\nавария плазматрон\nПлазматрон к заготовкед\nПлазматрон от заготовки\nПлазматрон к заготовке рабочее положение\nплазматро от заготовки рабочее положение\nБарабаны пуск\nБарабаны стоп\nПривод готов барабан 1\nавария привода барабана 1\nпитание включено барабаны\nбарабаны включены\nавария привода барабана 2\nпривод готов барабан 2\nПеремещение плазматрона пит. Включено\nempty\nПрижимной ролик вверху\nПрижимной ролик внизу\nempty", array type (2D Dbl)=string[] [] ("ОП1 Х1")) -> (array=→"ОП1 Х1 4":string[])
      n18 = Close File(refnum=w5, error in=w6) -> (path=w4:path, error out=w9:errorcluster)
      n19 = Unbundle(w9) -> ()  [unwired: 3 out]
    }
    frame #1 {
      n20 = while {
        tunnel: w62 -> [w89]
        stop <- FALSE stop-if-true
        w65 = "\t"
        n21 = Wait Until Next ms Multiple(millisecond multiple=u32 1000 ("milliseconds to wait")) -> ()  [unwired: 1 out]
        n22 = local read "Скорость ПП 2"() -> (w83:string)
        n23 = local read "ТЕМП КАМЕРА"() -> (w66:string)
        n24 = local read "V вращ. бараб"() -> (w84:string)
        n25 = local read "ТЕМП РОЛИК"() -> (w72:string)
        n26 = Get Date/Time In Seconds() -> (seconds since 1Jan1904=w98:timestamp)
        n27 = local read "Скорость ПП"() -> (w82:string)
        n28 = local read "ПОДШ. 1.1"() -> (w70:string)
        n29 = local read "ПОДШ. 1.2"() -> (w75:string)
        n30 = local read "ПОДШ. 2.1"() -> (w74:string)
        n31 = local read "ПОДШ. 2.2"() -> (w73:string)
        n32 = Format Date/Time String(seconds (now)=w98) -> (date/time string=w67:string)  [unwired: 2 in]
        n33 = local read "текущее значение\nзазора (mm)"() -> (w68:string)
        n34 = local read "U_ist"() -> (w81:string)
        n35 = local read "PT 1"() -> (w77:string)
        n36 = local read "PT 2"() -> (w76:string)
        n37 = local read "PT 3"() -> (w71:string)
        n38 = local read "PT 4"() -> (w64:string)
        n39 = local read "I_ist"() -> (w69:string)
        n40 = Open/Create/Replace File(file path (use dialog)=w89, error in=errorcluster {"status"=FALSE, "code"=0, "source"=""}) -> (refnum out=w97:refnum<file>, error out=w95:errorcluster)  [unwired: 4 in, 1 out]
        n41 = local read "PE1"() -> (w80:string)
        n42 = local read "PE2"() -> (w79:string)
        n43 = local read "PE3"() -> (w78:string)
        n44 = Concatenate Strings(w67, w65, w68, w65, w69, w65, w84, w65, w83, w65, w82, w65, w81, w65, w80, w65, w79, w65, w78, w65, w77, w65, w76, w65, w71, w65, w70, w65, w75, w65, w74, w65, w73, w65, w72, w65, w66, w65, w64, "\r") -> (w87:string)
        n45 = Set File Position(refnum=w97, from (0:start)=enum16{"start", "end", "current"}."end", error in=w95) -> (refnum out=w94:refnum<file>, error out=w93:errorcluster)  [unwired: 1 in]
        n46 = Write to Text File(file (use dialog)=w94, text=w87, error in=w93) -> (refnum out=w92:refnum<file>, error out=w91:errorcluster)  [unwired: 1 in, 1 out]
        n47 = Close File(refnum=w92, error in=w91) -> (error out=w90:errorcluster)  [unwired: 1 out]
        n48 = Unbundle(w90) -> ()  [unwired: 3 out]
      }
      n49 = while {
        stop <- FALSE stop-if-true
        w441 = i16 1 ("precision (6)")
        # "Вакуумная"
        n50 = local read "Y120"() -> (w580:bool[])
        n51 = local read "X200"() -> (w642:bool[])
        n52 = local read "X240"() -> (w626:bool[])
        n53 = local read "X100"() -> (w457:bool[])
        n54 = local read "X300"() -> (w601:bool[])
        n55 = local read "X340"() -> (w587:bool[])
        n56 = local read "X140"() -> (w661:bool[])
        n57 = local read "X400"() -> (w515:bool[])
        n58 = local read "Y60"() -> (w581:bool[])
        n59 = local read "out"() -> (→"Скорость толкателя":dbl)
        n60 = Get Date/Time In Seconds() -> (seconds since 1Jan1904=w524:timestamp)
        n61 = Wait Until Next ms Multiple(millisecond multiple=u32 500) -> ()  [unwired: 1 out]
        n62 = local read "V7045_U_ist"() -> (→"Напряжение":dbl)
        n63 = local read "V7045_I_ist"() -> (→"Ток":dbl)
        n64 = local read "PV_зазор"() -> (→"Значение зазора":dbl)
        n65 = local read "X140"() -> (w491:bool[])
        n66 = call "Метакон.vi"("Vak_in"="PT2") -> ("Vak_out_txt"=→"PT 2":string)  [unwired: 9 in, 1 out]
        n67 = call "Метакон.vi"("Vak_in"="PT3") -> ("Vak_out_txt"=→"PT 3":string)  [unwired: 9 in, 1 out]
        n68 = call "Метакон.vi"("Vak_in"="PT1") -> ("Vak_out_txt"=→"PT 1":string)  [unwired: 9 in, 1 out]
        n69 = Format Date/Time String(seconds (now)=w524) -> (date/time string=→"текущее время":string)  [unwired: 2 in]
        n70 = Number To Fractional String(number="Т1", precision (6)=w441) -> (F-format string=→"ПОДШ. 1.1":string)  [unwired: 2 in]
        n71 = Number To Fractional String(number="Т2", precision (6)=w441) -> (F-format string=→"ПОДШ. 1.2":string)  [unwired: 2 in]
        n72 = Number To Fractional String(number="Т3", precision (6)=w441) -> (F-format string=→"ПОДШ. 2.1":string)  [unwired: 2 in]
        n73 = Number To Fractional String(number="Т4", precision (6)=w441) -> (F-format string=→"ПОДШ. 2.2":string)  [unwired: 2 in]
        n74 = Number To Fractional String(number="Т5", precision (6)=w441) -> (F-format string=→"ТЕМП РОЛИК":string)  [unwired: 2 in]
        n75 = Number To Fractional String(number="Т6", precision (6)=w441) -> (F-format string=→"ТЕМП КАМЕРА":string)  [unwired: 2 in]
        n76 = call "presure PA.vi"("Volte"="PT3 2") -> ("presure String 2"=→"PT 4":string)  [unwired: 7 in, 3 out]
        n77 = Number To Boolean Array(number="x340") -> (Boolean array=w382:bool[])
        "X340" <- w382
        n78 = Number To Boolean Array(number="x200") -> (Boolean array=→"X200":bool[])
        n79 = Number To Boolean Array(number="x400") -> (Boolean array=→"X400":bool[])
        n80 = Number To Boolean Array(number="y120") -> (Boolean array=→"Y120":bool[])
        n81 = Number To Boolean Array(number="x140") -> (Boolean array=w377:bool[])
        "X140" <- w377
        n82 = Number To Boolean Array(number="x300") -> (Boolean array=→"X300":bool[])
        n83 = Number To Boolean Array(number="x240") -> (Boolean array=→"X240":bool[])
        n84 = Number To Boolean Array(number="x100") -> (Boolean array=w379:bool[])
        "X100" <- w379
        n85 = Number To Boolean Array(number="y60") -> (Boolean array=→"Y60":bool[])
        n86 = local read "V вращ. бараб"() -> (w548:string)
        n87 = local read "V барабаны 2"() -> (→"Частота вращения":dbl)
        n88 = Index Array(array=w587, index #1=2, index #2=5) -> ()  [unwired: 2 out]
        n89 = Number To Fractional String(number="PE3", precision (6)=i16 2) -> (F-format string=→"PE3" →"P камера (bar)":string)  [unwired: 2 in]
        n90 = Number To Fractional String(number="PE1", precision (6)=i16 2) -> (F-format string=→"PE1" →"P плазматрон (bar)":string)  [unwired: 2 in]
        n91 = Number To Fractional String(number="PE2", precision (6)=i16 1) -> (F-format string=→"PE2":string)  [unwired: 2 in]
        n92 = local read "Диаметр заг."() -> (w449:string)
        n93 = Index Array(array=w581, index #1=10, index #2=11, index #3=12) -> (element #1=w575:bool, element #2=w574:bool, element #3=w573:bool)
        n94 = Index Array(array=w515, index #1=18, index #2=29, index #3=30) -> (element #1=w519:bool, element #2=w521:bool, element #3=w522:bool)
        n95 = Index Array(array=w580, index #1=23, index #2=24, index #3=25, index #4=26) -> (element #1=w569:bool, element #2=w568:bool, element #3=w567:bool, element #4=w566:bool)
        n96 = Index Array(array=w661, index #1=16, index #2=18, index #3=19, index #4=20, index #5=21, index #6=24, index #7=25, index #8=28, index #9=29) -> (element #6=→"ролик_прижат":bool, element #7=→"ролик_отжат":bool, element #8=→"УГ_открыт":bool, element #9=→"УГ_закрыт":bool)  [unwired: 5 out]
        n97 = local read "U_ist"() -> (w543:string)
        n98 = To Long Integer(number="Скорость пп 2") -> (32bit integer=w446:i32)
        n99 = To Long Integer(number="Скорость пп") -> (32bit integer=w422:i32)
        n100 = Index Array(array=w642, index #1=1, index #2=6, index #3=7, index #4=27, index #5=14, index #6=13, index #7=21, index #8=22, index #9=23, index #10=24, index #11=25, index #12=19) -> ()  [unwired: 12 out]
        n101 = Index Array(array=w457, index #1=2, index #2=5, index #3=8, index #4=12, index #5=11, index #6=17, index #7=16, index #8=21, index #9=20, index #10=25, index #11=24, index #12=29, index #13=28) -> (element #1=w459:bool, element #2=w463:bool, element #3=w464:bool, element #4=w468:bool, element #5=w469:bool, element #6=w475:bool, element #7=w476:bool, element #8=w483:bool, element #9=w484:bool, element #10=w485:bool, element #11=w486:bool, element #12=w489:bool, element #13=w490:bool)
        n102 = Number To Fractional String(number="M_PLasmatron", precision (6)=i16 1) -> (F-format string=→"voto plasmatron":string)  [unwired: 2 in]
        n103 = Index Array(array=w626, index #1=16, index #2=17, index #3=18, index #4=19, index #5=20, index #6=9, index #7=12, index #8=13, index #9=16, index #10=17, index #11=18, index #12=19, index #13=21, index #14=22, index #15=23, index #16=27, index #17=28, index #18=29) -> (element #1=→"Air":bool, element #2=→"Air 4":bool, element #3=→"давление 1":bool, element #4=→"давление 2":bool)  [unwired: 14 out]
        n104 = Index Array(array=w601, index #1=0, index #2=1, index #3=8, index #4=9, index #5=12, index #6=13, index #7=20, index #8=21, index #9=22, index #10=23, index #11=24, index #12=25, index #13=26, index #14=27, index #15=28, index #16=29, index #17=30, index #18=31) -> (element #7=w600:bool, element #8=w599:bool, element #9=w598:bool, element #10=w597:bool, element #11=w596:bool, element #12=w595:bool, element #13=w594:bool, element #14=w593:bool, element #15=w592:bool, element #16=w591:bool, element #17=w590:bool)  [unwired: 7 out]
        n105 = Index Array(array=w491, index #1=4, index #2=5, index #3=6, index #4=9, index #5=8, index #6=11, index #7=10) -> (element #1=w502:bool, element #2=w503:bool, element #3=w504:bool, element #4=w375:bool, element #5=w374:bool, element #6=w372:bool, element #7=w373:bool)
        n106 = call "Индекс картинки.vi"("off"=w522, "on"=w521) -> ()  [unwired: 9 in, 1 out]
        n107 = Decimal String To Number(string=w543) -> (number=w542:i32)  [unwired: 2 in, 1 out]
        n108 = Decimal String To Number(string=w548) -> (number=w547:i32)  [unwired: 2 in, 1 out]
        n109 = Boolean To (0,1)(Boolean=w575) -> (0, 1=→"EV1":i16)
        n110 = Boolean To (0,1)(Boolean=w574) -> (0, 1=→"EV2":i16)
        n111 = Boolean To (0,1)(Boolean=w569) -> (0, 1=→"CO1":i16)
        n112 = Boolean To (0,1)(Boolean=w568) -> (0, 1=→"CO2":i16)
        n113 = Boolean To (0,1)(Boolean=w567) -> (0, 1=→"CO3":i16)
        n114 = Boolean To (0,1)(Boolean=w566) -> (0, 1=→"P1":i16)
        n115 = Decimal String To Number(string=w449) -> (number=w412:i32)  [unwired: 2 in, 1 out]
        n116 = Boolean To (0,1)(Boolean=w519) -> (0, 1=→"NL2":i16)
        n117 = Number To Decimal String(number=w446) -> (decimal integer string=w448:string)  [unwired: 1 in]
        n118 = Number To Decimal String(number=w422) -> (decimal integer string=w423:string)  [unwired: 1 in]
        n119 = Boolean To (0,1)(Boolean=w573) -> (0, 1=→"EV3.2" →"EV3.3" →"EV3.1":i16)
        n120 = Number To Fractional String(number="V барабаны задание", precision (6)=i16 0) -> (F-format string=→"V задания":string)  [unwired: 2 in]
        n121 = Multiply(x="ЗАДАНИЕ ТОКА", y=1.638) -> (x*y=w426:dbl)
        n122 = local read "Boolean"() -> (w402:bool)
        n123 = call "Индекс картинки.vi"("off"=w469, "on"=w468) -> ("index_image"=→"VP1":u16)  [unwired: 9 in]
        n124 = call "Индекс картинки.vi"("off"=w476, "on"=w475) -> ("index_image"=→"VP2":u16)  [unwired: 9 in]
        n125 = call "Индекс картинки.vi"("off"=w484, "on"=w483) -> ("index_image"=→"VP3":u16)  [unwired: 9 in]
        n126 = call "Индекс картинки.vi"("off"=w486, "on"=w485) -> ("index_image"=→"VP4":u16)  [unwired: 9 in]
        n127 = call "Индекс картинки.vi"("off"=w490, "on"=w489) -> ("index_image"=→"VP5":u16)  [unwired: 9 in]
        n128 = call "Индекс картинки.vi"("off"=w374, "on"=w375) -> ("index_image"=→"PD1":u16)  [unwired: 9 in]
        n129 = call "Индекс картинки.vi"("off"=w373, "on"=w372) -> ("index_image"=→"PD2":u16)  [unwired: 9 in]
        n130 = local write "Скорость ПП 2"(w448) -> ()
        n131 = local write "Скорость ПП"(w423) -> ()
        n132 = Index Array(array=w382, index=4) -> (element=→"Газ":bool)
        n133 = Boolean To (0,1)(Boolean=w459) -> (0, 1=→"NL1":i16)
        n134 = Boolean To (0,1)(Boolean=w464) -> (0, 1=→"NR1":i16)
        n135 = Boolean To (0,1)(Boolean=w463) -> (0, 1=→"NZ1":i16)
        n136 = Boolean To (0,1)(Boolean=w504) -> (0, 1=→"PT3":i16)
        n137 = Boolean To (0,1)(Boolean=w502) -> (0, 1=→"PT1":i16)
        n138 = Boolean To (0,1)(Boolean=w503) -> (0, 1=→"PT2":i16)
        n139 = Index Array(array=w377, index=17) -> (element=→"Распыление":bool)
        n140 = Equal?(x=w412, y=0) -> (x = y?=w415:bool)
        n141 = Greater Or Equal?(x=w542, y=20) -> (x >= y?=w540:bool)
        n142 = Greater Or Equal?(x=w547, y=500) -> (x >= y?=w545:bool)
        n143 = Index Array(array=w379, index=1) -> (element=→"Вакуум":bool)
        n144 = call "Метакон.vi"("Vak_in"="PT4") -> ("Vak_out_txt"=→"PT 4txt":string)  [unwired: 9 in, 1 out]
        n145 = Build Array(w600, w599, w598, w597, w596, w595, w594, w593, w592, w591, w590) -> (w386:bool[])
        n146 = property on="Arhive" class="Bool"() -> ("DisabledEnum"=w400:T7)  [unwired: 2 in, 2 out]
        n147 = And(x=w540, y=w545) -> (x .and. y?=w544:bool)
        n148 = To Long Integer(number=w426) -> (32bit integer=w427:i32)
        n149 = local write "Запись отчета"(w544) -> ()
        n150 = Number To Decimal String(number=w427) -> (decimal integer string=w428:string)  [unwired: 1 in]
        n151 = Not Equal?(x=w400, y=T7."Disabled and Grayed Out" ("Disabled")) -> (x != y?=w404:bool)
        n152 = Not Equal?(x=w400, y=T7."Enabled") -> (x != y?=w398:bool)
        n153 = case shown="False" w415 {
          tunnel: w412 -> [w664 _]
          tunnel: [w664 210] -> w411
          frame False {
          }
          frame True {
          }
        }
        n154 = And(x=w402, y=w404) -> (x .and. y?=w405:bool)
        n155 = case shown="True" w405 {
          frame False {
          }
          frame True {
            n156 = property on="Arhive" class="Bool"("DisabledEnum"=T7."Disabled and Grayed Out" ("Disabled")) -> ()  [unwired: 2 in, 2 out]
          }
        }
        n157 = call "4.2 индикар полки.vi"("appended array"=w386) -> ("текущее положение"=→"ИНдикатор положения полки":string)  [unwired: 10 in]
        n158 = Not(x=w402) -> (.not. x?=w401:bool)
        n159 = And(x=w401, y=w398) -> (x .and. y?=w397:bool)
        n160 = local write "задание тока А"(w428) -> ()
        n161 = Number To Decimal String(number="V5014") -> (decimal integer string=w387:string)  [unwired: 1 in]
        n162 = case shown="True" w397 {
          frame False {
          }
          frame True {
            n163 = property on="Arhive" class="Bool"("DisabledEnum"=T7."Enabled" ("Disabled")) -> ()  [unwired: 2 in, 2 out]
          }
        }
        n164 = local write "Пауза допыления"(w387) -> ()
        n165 = Divide(x=210.0, y=w411) -> (x/y=w409:dbl)
        n166 = Multiply(x=9180, y=w409) -> (x*y=w407:dbl)
        n167 = Number To Fractional String(number=w407, precision (6)=i16 0) -> (F-format string=→"max Speed":string)  [unwired: 2 in]
        n168 = Multiply(x="V барабаны", y=w409) -> (x*y=w453:dbl)
        n169 = To Long Integer(number=w453) -> (32bit integer=w414:i32)
        "V барабаны 2" <- w414
        n170 = Number To Fractional String(number=w414, precision (6)=i16 0) -> (F-format string=→"V вращ. бараб":string)  [unwired: 2 in]
        "PT4 2" <- u16 1 ("PT4")
      }
      n171 = while {
        stop <- FALSE stop-if-true
        n172 = event shown="[28] \"напустить газ в камеру\": Value Change" {
          selector: _ -> [_ _ _ _ _ _ _ _ _ _ _ _ _ _ _ _ _ _ _ _ _ _ _ _ _ _ _ _ _ _ _ _]
          dyn-events: _ -> [_ _ _ _ _ _ _ _ _ _ _ _ _ _ _ _ _ _ _ _ _ _ _ _ _ _ _ _ _ _ _ _]
          timeout: _ -> [_ _ _ _ _ _ _ _ _ _ _ _ _ _ _ _ _ _ _ _ _ _ _ _ _ _ _ _ _ _ _ _]
          event "Выход": Value Change {
            n173 = event-data() -> ()  [unwired: 1 in, 5 out]
            n174 = Stop(stop? (T)="Выход") -> ()
          }
          event "Arhive": Value Change {
            n175 = event-data() -> ()  [unwired: 1 in, 5 out]
            n176 = call "3.1.форма базы отчетов_UCRI.vi"() -> ()  [unwired: 12 in]
          }
          event "Сохранить настройки": Value Change {
            w148 = i16 0 ("precision (6)")
            n177 = event-data() -> ()  [unwired: 1 in, 5 out]
            n178 = local read "Параметры измерения"() -> (w188:T3)
            n179 = local read "Индикатор камеры 2"() -> (w171:bool)
            n180 = local read "Индикатор камеры"() -> (w198:bool)
            n181 = local read "Уровень бинаризации"() -> (w174:T4)
            n182 = local read "Область измерения"() -> (w197:T2)
            n183 = Unbundle(w188) -> ("Contrast"=w187:i32, "Filter width"=w186:i32, "Steepness"=w185:i32, "Subsampling Ratio"=w184:u32, "Show Search Area"=w183:bool, "Show Search Lines"=w182:bool, "Show Edges Found"=w181:bool, "Show Result"=w180:bool)
            n184 = local read "Рабочий цвет"() -> (w139:u32)
            n185 = local read "Калибровка"() -> (w175:u32)
            n186 = local read "Задержка"() -> (w196:u32)
            n187 = call <vilib>:"Application Directory.vi"() -> ("Application Directory"=w144:path)
            n188 = local read "Фильтр"() -> (w194:i32)
            n189 = Unbundle(w174) -> ("Нижний предел"=w173:sgl, "Верхний предел"=w172:sgl)
            n190 = Boolean To (0,1)(Boolean=w198) -> (0, 1=w195:i16)
            n191 = Boolean To (0,1)(Boolean=w183) -> (0, 1=w179:i16)
            n192 = Boolean To (0,1)(Boolean=w182) -> (0, 1=w178:i16)
            n193 = Boolean To (0,1)(Boolean=w181) -> (0, 1=w177:i16)
            n194 = Boolean To (0,1)(Boolean=w180) -> (0, 1=w176:i16)
            n195 = Boolean To (0,1)(Boolean=w171) -> (0, 1=w151:i16)
            n196 = Unbundle(w197) -> ("Left"=w193:i32, "Top"=w192:i32, "Right"=w191:i32, "Bottom"=w190:i32, "Rotation"=w189:dbl)
            n197 = Path To String(path=w144) -> (string=w143:string)
            n198 = Number To Fractional String(number=w179, precision (6)=w148) -> (F-format string=w158:string)  [unwired: 2 in]
            n199 = Number To Fractional String(number=w178, precision (6)=w148) -> (F-format string=w157:string)  [unwired: 2 in]
            n200 = Number To Fractional String(number=w177, precision (6)=w148) -> (F-format string=w156:string)  [unwired: 2 in]
            n201 = Number To Fractional String(number=w176, precision (6)=w148) -> (F-format string=w155:string)  [unwired: 2 in]
            n202 = Number To Fractional String(number=w196) -> (F-format string=w169:string)  [unwired: 3 in]
            n203 = Number To Fractional String(number=w194) -> (F-format string=w168:string)  [unwired: 3 in]
            n204 = Number To Fractional String(number=w193) -> (F-format string=w167:string)  [unwired: 3 in]
            n205 = Number To Fractional String(number=w192) -> (F-format string=w166:string)  [unwired: 3 in]
            n206 = Number To Fractional String(number=w191) -> (F-format string=w165:string)  [unwired: 3 in]
            n207 = Number To Fractional String(number=w190) -> (F-format string=w164:string)  [unwired: 3 in]
            n208 = Number To Fractional String(number=w189) -> (F-format string=w163:string)  [unwired: 3 in]
            n209 = Number To Fractional String(number=w187) -> (F-format string=w162:string)  [unwired: 3 in]
            n210 = Number To Fractional String(number=w186) -> (F-format string=w161:string)  [unwired: 3 in]
            n211 = Number To Fractional String(number=w185) -> (F-format string=w160:string)  [unwired: 3 in]
            n212 = Number To Fractional String(number=w184) -> (F-format string=w159:string)  [unwired: 3 in]
            n213 = Number To Fractional String(number=w175) -> (F-format string=w154:string)  [unwired: 3 in]
            n214 = Number To Fractional String(number=w173) -> (F-format string=w153:string)  [unwired: 3 in]
            n215 = Number To Fractional String(number=w172) -> (F-format string=w152:string)  [unwired: 3 in]
            n216 = Number To Fractional String(number=w195, precision (6)=i16 0) -> (F-format string=w170:string)  [unwired: 2 in]
            n217 = Number To Fractional String(number=w151, precision (6)=i16 0) -> (F-format string=w150:string)  [unwired: 2 in]
            n218 = Number To Fractional String(number=w139, precision (6)=i16 0) -> (F-format string=w137:string)  [unwired: 2 in]
            n219 = local read "Камера"() -> (w149:T1)
            n220 = Concatenate Strings(w143, "\\set_cam" ("string")) -> (w141:string)
            n221 = Build Array(w149, w170, w169, w168, w167, w166, w165, w164, w163, w162, w161, w160, w159, w158, w157, w156, w155, w154, w153, w152, w150, w137) -> (w145:T1[])
            n222 = String To Path(string=w141) -> (path=w140:path)
            n223 = call-poly <vilib>:"Write To Spreadsheet File.vi"("1D data"=w145, "file path (dialog if empty)"=w140) -> ()  [unwired: 6 in, 1 out]
          }
          event "V задания": Mouse Down {
            (unwired) "" ("ТЕКУЩЕЕ ЗНАЧЕНИЕ")
            n224 = event-data() -> ()  [unwired: 1 in, 7 out]
            n225 = local read "max Speed"() -> (w200:string)
            n226 = local read "V задания"() -> (w201:string)
            n227 = Decimal String To Number(string=w200) -> (number=w199:i32)  [unwired: 2 in, 1 out]
            n228 = call "NUMPAD1_9(ПРОГРАММА).vi"("МИНИМАЛЬНОЕ ЗНАЧЕНИЕ"=-1.0, "МАКСИМАЛЬНОЕ ЗНАЧЕНИЕ"=w199, "ДЛИННА СЛОВА"=i8 5, "ТЕКУЩЕЕ ЗНАЧЕНИЕ"=w201) -> ("НОВОЕ ЗНАЧЕНИЕ"=w203:string)  [unwired: 7 in]
            n229 = Fract/Exp String To Number(string=w203) -> (number=w202:dbl)  [unwired: 3 in, 1 out]
            n230 = DataSocket Write(8:errorcluster {"status"=FALSE, "code"=0, "source"=""} ("error in (no error)"), 9:500 ("ms timeout (0)"), 10:w202, 11:"opc://localhost/National Instruments.NIOPCServers/CNL_1.PLC1.PARAM_RASP.SP_S_MOVE" ("connection in")) -> ()  [unwired: 3 out]
          }
          event "Диаметр заг.": Mouse Down {
            n231 = event-data() -> ()  [unwired: 1 in, 7 out]
            n232 = local read "Диаметр заг."() -> (w209:string)
            n233 = call "NUMPAD1_9.vi"("МИНИМАЛЬНОЕ ЗНАЧЕНИЕ"=40.0, "МАКСИМАЛЬНОЕ ЗНАЧЕНИЕ"=90.0, "ДЛИННА СЛОВА"=i8 2, "ТЕКУЩЕЕ ЗНАЧЕНИЕ"=w209) -> ("НОВОЕ ЗНАЧЕНИЕ"=w214:string)  [unwired: 7 in]
            n234 = Fract/Exp String To Number(string=w214) -> (number=w213:dbl)  [unwired: 3 in, 1 out]
            n235 = Multiply(x=w213, y=10.0) -> (x*y=w211:dbl)
            n236 = To Word Integer(number=w211) -> (16bit integer=w210:i16)
            n237 = DataSocket Write(8:errorcluster {"status"=FALSE, "code"=0, "source"=""} ("error in (no error)"), 9:100 ("ms timeout (0)"), 10:w210, 11:"opc://localhost/National Instruments.NIOPCServers/CNL_1.PLC1.PARAM_RASP.D_ZAG") -> (0:w216:errorcluster)  [unwired: 2 out]
            n238 = Unbundle(w216) -> ()  [unwired: 3 out]
          }
          event "ГС -Открыть": Value Change {
            n239 = event-data() -> ()  [unwired: 1 in, 5 out]
            n240 = DataSocket Write(8:errorcluster {"status"=FALSE, "code"=0, "source"=""} ("error in (no error)"), 9:500 ("ms timeout (0)"), 10:TRUE, 11:"" ("connection in")) -> ()  [unwired: 3 out]
          }
          event "ГС - Закрыть": Value Change {
            n241 = event-data() -> ()  [unwired: 1 in, 5 out]
            n242 = DataSocket Write(8:errorcluster {"status"=FALSE, "code"=0, "source"=""} ("error in (no error)"), 9:500 ("ms timeout (0)"), 10:TRUE, 11:"" ("connection in")) -> ()  [unwired: 3 out]
          }
          event "Продол назад": Value Change {
            n243 = event-data() -> ()  [unwired: 1 in, 5 out]
            n244 = DataSocket Write(8:errorcluster {"status"=FALSE, "code"=0, "source"=""} ("error in (no error)"), 9:500 ("ms timeout (0)"), 10:TRUE, 11:"opc://localhost/National Instruments.NIOPCServers/CNL_1.PLC1.Makro.c601" ("connection in")) -> ()  [unwired: 3 out]
          }
          event "Продол впер": Value Change {
            n245 = event-data() -> ()  [unwired: 1 in, 5 out]
            n246 = local read "Порядковый номер"() -> (w237:string)
            n247 = Decimal String To Number(string=w237) -> (number=w236:i32)  [unwired: 2 in, 1 out]
            n248 = Increment(x=w236) -> (x+1=w235:i32)
            n249 = Number To Decimal String(number=w235) -> (decimal integer string=w234:string)  [unwired: 1 in]
            n250 = local write "Порядковый номер"(w234) -> ()
            n251 = DataSocket Write(8:errorcluster {"status"=FALSE, "code"=0, "source"=""} ("error in (no error)"), 9:500 ("ms timeout (0)"), 10:TRUE, 11:"opc://localhost/National Instruments.NIOPCServers/CNL_1.PLC1.Makro.c602" ("connection in")) -> ()  [unwired: 3 out]
          }
          event "ПОДАЧА ЗАГОТОВКИ": Value Change {
            n252 = event-data() -> ()  [unwired: 1 in, 5 out]
            n253 = DataSocket Write(8:errorcluster {"status"=FALSE, "code"=0, "source"=""} ("error in (no error)"), 9:250 ("ms timeout (0)"), 10:TRUE, 11:"opc://localhost/National Instruments.NIOPCServers/DL.DL260.Buttons.Заг-набар" ("connection in")) -> (0:w242:errorcluster)  [unwired: 2 out]
            n254 = Unbundle(w242) -> ()  [unwired: 3 out]
          }
          event "Автораспыление доплавить": Value Change {
            n255 = event-data() -> ()  [unwired: 1 in, 5 out]
          }
          event "Автораспыление начать": Value Change {
            n256 = event-data() -> ()  [unwired: 1 in, 5 out]
            n257 = DataSocket Write(8:errorcluster {"status"=FALSE, "code"=0, "source"=""} ("error in (no error)"), 9:250 ("ms timeout (0)"), 10:TRUE, 11:"opc://localhost/National Instruments.NIOPCServers/DL.DL260.Buttons.расплав-начать" ("connection in")) -> ()  [unwired: 3 out]
          }
          event "ПЛАЗМАТРОН В ИСХОДНОЕ": Value Change {
            n258 = event-data() -> ()  [unwired: 1 in, 5 out]
            n259 = DataSocket Write(8:errorcluster {"status"=FALSE, "code"=0, "source"=""} ("error in (no error)"), 9:500 ("ms timeout (0)"), 10:TRUE, 11:"opc://localhost/National Instruments.NIOPCServers/CNL_1.PLC1.Makro.c600" ("connection in")) -> ()  [unwired: 3 out]
          }
          event "Закончить автораспыление": Value Change {
            n260 = event-data() -> ()  [unwired: 1 in, 5 out]
            n261 = DataSocket Write(8:errorcluster {"status"=FALSE, "code"=0, "source"=""} ("error in (no error)"), 9:250 ("ms timeout (0)"), 10:TRUE, 11:"opc://localhost/National Instruments.NIOPCServers/DL.DL260.Buttons.расплав-закончить" ("connection in")) -> ()  [unwired: 3 out]
          }
          event "Скорость ПП": Mouse Down {
            n262 = event-data() -> ()  [unwired: 1 in, 7 out]
            n263 = call "NUMPAD1_9.vi"("МИНИМАЛЬНОЕ ЗНАЧЕНИЕ"=0.0, "МАКСИМАЛЬНОЕ ЗНАЧЕНИЕ"=601.0, "ДЛИННА СЛОВА"=i8 3, "ТЕКУЩЕЕ ЗНАЧЕНИЕ"="Скорость ПП") -> ("НОВОЕ ЗНАЧЕНИЕ"=w267:string)  [unwired: 7 in]
            n264 = Decimal String To Number(string=w267) -> (number=w259:i32)  [unwired: 2 in, 1 out]
            n265 = To Long Integer(number=w259) -> (32bit integer=w260:i32)
            n266 = DataSocket Write(8:errorcluster {"status"=FALSE, "code"=0, "source"=""} ("error in (no error)"), 9:250 ("ms timeout (0)"), 10:w260, 11:"opc://localhost/National Instruments.NIOPCServers/CNL_1.PLC1.PARAM_RASP.OUT_P_SAG_M" ("connection in")) -> ()  [unwired: 3 out]
            n267 = DataSocket Write(8:errorcluster {"status"=FALSE, "code"=0, "source"=""} ("error in (no error)"), 9:250 ("ms timeout (0)"), 10:w260, 11:"opc://localhost/National Instruments.NIOPCServers/CNL_1.PLC1.PARAM_RASP.4165" ("connection in")) -> ()  [unwired: 3 out]
          }
          event "Скорость ПП 2": Mouse Down {
            n268 = event-data() -> ()  [unwired: 1 in, 7 out]
            n269 = call "NUMPAD1_9.vi"("МИНИМАЛЬНОЕ ЗНАЧЕНИЕ"=0.0, "МАКСИМАЛЬНОЕ ЗНАЧЕНИЕ"=361.0, "ДЛИННА СЛОВА"=i8 3, "ТЕКУЩЕЕ ЗНАЧЕНИЕ"="Скорость ПП 2") -> ("НОВОЕ ЗНАЧЕНИЕ"=w281:string)  [unwired: 7 in]
            n270 = Decimal String To Number(string=w281) -> (number=w273:i32)  [unwired: 2 in, 1 out]
            n271 = To Long Integer(number=w273) -> (32bit integer=w274:i32)
            n272 = DataSocket Write(8:errorcluster {"status"=FALSE, "code"=0, "source"=""} ("error in (no error)"), 9:250 ("ms timeout (0)"), 10:w274, 11:"opc://localhost/National Instruments.NIOPCServers/CNL_1.PLC1.PARAM_RASP.SP_PR_PLAZM" ("connection in")) -> ()  [unwired: 3 out]
            n273 = DataSocket Write(8:errorcluster {"status"=FALSE, "code"=0, "source"=""} ("error in (no error)"), 9:250 ("ms timeout (0)"), 10:w274, 11:"opc://localhost/National Instruments.NIOPCServers/CNL_1.PLC1.PARAM_RASP.4166" ("connection in")) -> ()  [unwired: 3 out]
          }
          event "Пауза допыления": Mouse Down {
            n274 = event-data() -> ()  [unwired: 1 in, 7 out]
            n275 = call "NUMPAD1_9.vi"("МИНИМАЛЬНОЕ ЗНАЧЕНИЕ"=-1.0, "МАКСИМАЛЬНОЕ ЗНАЧЕНИЕ"=10.0, "ДЛИННА СЛОВА"=i8 1, "ТЕКУЩЕЕ ЗНАЧЕНИЕ"="Пауза допыления") -> ("НОВОЕ ЗНАЧЕНИЕ"=w289:string)  [unwired: 7 in]
            n276 = Decimal String To Number(string=w289) -> (number=w288:i32)  [unwired: 2 in, 1 out]
            n277 = DataSocket Write(8:errorcluster {"status"=FALSE, "code"=0, "source"=""} ("error in (no error)"), 9:250 ("ms timeout (0)"), 10:w288, 11:"opc://localhost/National Instruments.NIOPCServers/CNL_1.PLC1.RID.V5014") -> (0:w285:errorcluster)  [unwired: 2 out]
            n278 = Unbundle(w285) -> ()  [unwired: 3 out]
          }
          event "автоматическое включение регулятора": Value Change {
            n279 = event-data() -> ()  [unwired: 1 in, 5 out]
            n280 = DataSocket Write(8:errorcluster {"status"=FALSE, "code"=0, "source"=""} ("error in (no error)"), 9:500 ("ms timeout (0)"), 10:TRUE (".not. x?"), 11:"opc://localhost/National Instruments.NIOPCServers/CNL_1.PLC1.RID.C23") -> (0:w298:errorcluster)  [unwired: 2 out]
            n281 = Unbundle(w298) -> ()  [unwired: 3 out]
          }
          event "МАКСИМАЛЬНАЯ СКОРОСТЬ ПП К": Value Change {
            w300 = "opc://localhost/National Instruments.NIOPCServers/CNL_1.PLC1.PARAM_RASP.SP_PR_PLAZM"  # opc://localhost/National Instruments.NIOPCServers/CNL_1.PLC1.PARAM_RASP.SP_PR_PLAZM
            w304 = "opc://localhost/National Instruments.NIOPCServers/CNL_1.PLC1.PARAM_RASP.SP_PR_ZAG"  # opc://localhost/National Instruments.NIOPCServers/CNL_1.PLC1.PARAM_RASP.SP_PR_ZAG
            n282 = event-data() -> ()  [unwired: 1 in, 5 out]
            n283 = DataSocket Write(8:errorcluster {"status"=FALSE, "code"=0, "source"=""} ("error in (no error)"), 10:600, 11:w304) -> ()  [unwired: 1 in, 3 out]
            n284 = DataSocket Write(8:errorcluster {"status"=FALSE, "code"=0, "source"=""} ("error in (no error)"), 10:360, 11:w300) -> ()  [unwired: 1 in, 3 out]
          }
          event "задание тока А": Mouse Down {
            n285 = event-data() -> ()  [unwired: 1 in, 7 out]
            n286 = call "NUMPAD1_9.vi"("МИНИМАЛЬНОЕ ЗНАЧЕНИЕ"=0.0, "МАКСИМАЛЬНОЕ ЗНАЧЕНИЕ"=2500.0, "ДЛИННА СЛОВА"=i8 4, "ТЕКУЩЕЕ ЗНАЧЕНИЕ"="задание тока А") -> ("НОВОЕ ЗНАЧЕНИЕ"=w314:string)  [unwired: 7 in]
            n287 = Decimal String To Number(string=w314) -> (number=w313:i32)  [unwired: 2 in, 1 out]
            n288 = Multiply(x=w313, y=1.638) -> (x*y=w311:dbl)
            n289 = To Long Integer(number=w311) -> (32bit integer=w310:i32)
            n290 = DataSocket Write(8:errorcluster {"status"=FALSE, "code"=0, "source"=""} ("error in (no error)"), 9:250 ("ms timeout (0)"), 10:w310, 11:"opc://localhost/National Instruments.NIOPCServers/DL.DL260.Vmem.ист-задание" ("connection in")) -> ()  [unwired: 3 out]
          }
          event "Улавливатель закрыть": Value Change {
            n291 = event-data() -> ()  [unwired: 1 in, 5 out]
          }
          event "Улавливатель открыть": Value Change {
            n292 = event-data() -> ()  [unwired: 1 in, 5 out]
          }
          event "Ролик прижать": Value Change {
            n293 = event-data() -> ()  [unwired: 1 in, 5 out]
            n294 = DataSocket Write(8:errorcluster {"status"=FALSE, "code"=0, "source"=""} ("error in (no error)"), 9:500 ("ms timeout (0)"), 10:TRUE, 11:"opc://localhost/National Instruments.NIOPCServers/DL.DL260.Buttons.Рол-прижать" ("connection in")) -> ()  [unwired: 3 out]
          }
          event "Ролик отжать": Value Change {
            n295 = event-data() -> ()  [unwired: 1 in, 5 out]
            n296 = DataSocket Write(8:errorcluster {"status"=FALSE, "code"=0, "source"=""} ("error in (no error)"), 9:500 ("ms timeout (0)"), 10:TRUE, 11:"opc://localhost/National Instruments.NIOPCServers/DL.DL260.Buttons.Рол-отжать" ("connection in")) -> ()  [unwired: 3 out]
          }
          event "откачать рабочий вакуум": Value Change {
            n297 = event-data() -> ()  [unwired: 1 in, 5 out]
            n298 = property on="откачать рабочий вакуум" class="Bool"() -> ("BoolText.Text"=w331:string)  [unwired: 2 in, 2 out]
            n299 = call "Диалог_на_Макро.vi"("СОСТОЯНИЕ"="mac 2", "String"=w331) -> ("ВЫХОД"=w327:bool)  [unwired: 9 in]
            n300 = DataSocket Write(9:500 ("ms timeout (0)"), 10:w327, 11:"opc://localhost/National Instruments.NIOPCServers/CNL_1.PLC1.Makro.c200" ("connection in")) -> (0:w330:errorcluster)  [unwired: 1 in, 2 out]
            n301 = Unbundle(w330) -> ()  [unwired: 3 out]
          }
          event "forvacuum": Value Change {
            n302 = event-data() -> ()  [unwired: 1 in, 5 out]
            n303 = property on="forvacuum" class="Bool"() -> ("BoolText.Text"=w332:string)  [unwired: 2 in, 2 out]
            n304 = call "Диалог_на_Макро.vi"("СОСТОЯНИЕ"="forvakuum led", "String"=w332) -> ("ВЫХОД"=w337:bool)  [unwired: 9 in]
            n305 = DataSocket Write(9:500 ("ms timeout (0)"), 10:w337, 11:"opc://localhost/National Instruments.NIOPCServers/CNL_1.PLC1.Makro.c251" ("connection in")) -> (0:w334:errorcluster)  [unwired: 1 in, 2 out]
            n306 = Unbundle(w334) -> ()  [unwired: 3 out]
          }
          event "ND HEAT BUT": Value Change {
            n307 = event-data() -> ()  [unwired: 1 in, 5 out]
            n308 = property on="ND HEAT BUT" class="Bool"() -> ("BoolText.Text"=w338:string)  [unwired: 2 in, 2 out]
            n309 = call "Диалог_на_Макро.vi"("СОСТОЯНИЕ"="ND HEAT LED", "String"=w338) -> ("ВЫХОД"=w343:bool)  [unwired: 9 in]
            n310 = DataSocket Write(9:500 ("ms timeout (0)"), 10:w343, 11:"opc://localhost/National Instruments.NIOPCServers/CNL_1.PLC1.Makro.c250" ("connection in")) -> (0:w340:errorcluster)  [unwired: 1 in, 2 out]
            n311 = Unbundle(w340) -> ()  [unwired: 3 out]
          }
          event "откачка стоп": Value Change {
            n312 = event-data() -> ()  [unwired: 1 in, 5 out]
            n313 = property on="откачка стоп" class="Bool"() -> ("BoolText.Text"=w344:string)  [unwired: 2 in, 2 out]
            n314 = call "Диалог_на_Макро.vi"("СОСТОЯНИЕ"="mac3", "String"=w344) -> ("ВЫХОД"=w346:bool)  [unwired: 9 in]
            n315 = DataSocket Write(9:500 ("ms timeout (0)"), 10:w346, 11:"opc://localhost/National Instruments.NIOPCServers/CNL_1.PLC1.Makro.c201" ("connection in")) -> (0:w349:errorcluster)  [unwired: 1 in, 2 out]
            n316 = Unbundle(w349) -> ()  [unwired: 3 out]
          }
          event "напустить газ в камеру": Value Change {
            n317 = event-data() -> ()  [unwired: 1 in, 5 out]
            n318 = property on="напустить газ в камеру" class="Bool"() -> ("BoolText.Text"=w355:string)  [unwired: 2 in, 2 out]
            n319 = call "Диалог_на_Макро.vi"("СОСТОЯНИЕ"="mac 4", "String"=w355) -> ("ВЫХОД"=w350:bool)  [unwired: 9 in]
            n320 = DataSocket Write(9:500 ("ms timeout (0)"), 10:w350, 11:"opc://localhost/National Instruments.NIOPCServers/CNL_1.PLC1.Makro.napusk" ("connection in")) -> (0:w353:errorcluster)  [unwired: 1 in, 2 out]
            n321 = Unbundle(w353) -> ()  [unwired: 3 out]
          }
          event "напустить гелий в ресивер": Value Change {
            n322 = event-data() -> ()  [unwired: 1 in, 5 out]
            n323 = property on="напустить гелий в ресивер" class="Bool"() -> ("BoolText.Text"=w356:string)  [unwired: 2 in, 2 out]
            n324 = call "Диалог_на_Макро.vi"("СОСТОЯНИЕ"="mac5", "String"=w356) -> ("ВЫХОД"=w359:bool)  [unwired: 9 in]
            n325 = DataSocket Write(9:500 ("ms timeout (0)"), 10:w359, 11:"opc://localhost/National Instruments.NIOPCServers/CNL_1.PLC1.Makro.C610") -> (0:w361:errorcluster)  [unwired: 1 in, 2 out]
            n326 = Unbundle(w361) -> ()  [unwired: 3 out]
          }
          event "напустить аргон в ресивер": Value Change {
            n327 = event-data() -> ()  [unwired: 1 in, 5 out]
            n328 = property on="напустить аргон в ресивер" class="Bool"() -> ("BoolText.Text"=w362:string)  [unwired: 2 in, 2 out]
            n329 = call "Диалог_на_Макро.vi"("СОСТОЯНИЕ"="mac6", "String"=w362) -> ("ВЫХОД"=w365:bool)  [unwired: 9 in]
            n330 = DataSocket Write(9:500 ("ms timeout (0)"), 10:w365, 11:"opc://localhost/National Instruments.NIOPCServers/CNL_1.PLC1.Makro.C611") -> (0:w367:errorcluster)  [unwired: 1 in, 2 out]
            n331 = Unbundle(w367) -> ()  [unwired: 3 out]
          }
          event "ЗУ-вверх": Value Change {
            n332 = event-data() -> ()  [unwired: 1 in, 5 out]
            n333 = DataSocket Write(8:errorcluster {"status"=FALSE, "code"=0, "source"=""} ("error in (no error)"), 9:500 ("ms timeout (0)"), 10:TRUE, 11:"opc://localhost/National Instruments.NIOPCServers/CNL_1.PLC1.Makro.s226" ("connection in")) -> ()  [unwired: 3 out]
          }
        }
        n334 = Wait Until Next ms Multiple(millisecond multiple=u32 500) -> ()  [unwired: 1 out]
      }
      n335 = while {
        stop <- FALSE stop-if-true
        n336 = Get Date/Time In Seconds() -> (seconds since 1Jan1904=w105:timestamp)
        n337 = Wait (ms)(milliseconds to wait=u32 500) -> ()  [unwired: 1 out]
        n338 = Format Date/Time String(seconds (now)=w105) -> (date/time string=w99:string)  [unwired: 2 in]
        n339 = Greater?(x="Ошибка 2", y=i16 0) -> (0:w101:bool)
        n340 = case shown="True" w101 {
          tunnel: "Ошибка 2" -> [_ w108]
          tunnel: w99 -> [_ w116]
          frame False {
          }
          frame True {
            w110 = "\r"
            w118 = "\t"
            n341 = call "4.1. описание ошибки.vi"("Numeric"=w108) -> ("String 2"=w106:string, "String"=w107:string)  [unwired: 9 in]
            n342 = local write "Ошибка 2"(i16 0 ("Ошибка 2")) -> ()
            n343 = Number To Decimal String(number=w108) -> (decimal integer string=w114:string)  [unwired: 1 in]
            n344 = call "путь для общего отчета.vi"() -> ("path_out 2"=w119:string)  [unwired: 11 in]
            n345 = Concatenate Strings(w116, w118, w114, w118, w107, "   " ("string"), w106, "\n") -> (w120:string)
            n346 = Concatenate Strings("Data: " ("string"), w116, w110, "Numer: " ("string"), w114, w110, w107, w110, w106) -> (w113:string)
            n347 = Concatenate Strings(w119, "errors.txt") -> (w131:string)
            n348 = call "2.6. форма ошибки.vi"("Описание ошибки"=w113) -> ()  [unwired: 11 in]
            n349 = String To Path(string=w131) -> (path=w133:path)
            n350 = Open/Create/Replace File(file path (use dialog)=w133, error in=errorcluster {"status"=FALSE, "code"=0, "source"=""}, operation (0:open)=T6."open or create") -> (refnum out=w126:refnum<file>, error out=w128:errorcluster)  [unwired: 3 in, 1 out]
            n351 = Set File Position(refnum=w126, from (0:start)=enum16{"start", "end", "current"}."end", error in=w128) -> (refnum out=w124:refnum<file>, error out=w125:errorcluster)  [unwired: 1 in]
            n352 = Write to Text File(file (use dialog)=w124, text=w120, error in=w125) -> (refnum out=w123:refnum<file>, error out=w122:errorcluster)  [unwired: 1 in, 1 out]
            n353 = Close File(refnum=w123, error in=w122) -> (error out=w121:errorcluster)  [unwired: 1 out]
            n354 = Unbundle(w121) -> ()  [unwired: 3 out]
          }
        }
      }
    }
  }
  n355 = while {
    stop <- "stop 2" stop-if-true
    n356 = Wait Until Next ms Multiple(millisecond multiple=u32 250) -> ()  [unwired: 1 out]
    n357 = event shown="[13] \"откачка стоп 2\": Value Change" {
      selector: _ -> [_ _ _ _ _ _ _ _ _ _ _ _ _ _]
      dyn-events: _ -> [_ _ _ _ _ _ _ _ _ _ _ _ _ _]
      timeout: 250 -> [_ _ _ _ _ _ _ _ _ _ _ _ _ _]
      event Timeout {
        n358 = event-data() -> ()  [unwired: 1 in, 2 out]
        n359 = local read "D, заготовки"() -> (w694:i16)
        n360 = Number To Decimal String(number="max out") -> (decimal integer string=→"Максимальная подача (мм/мин)2":string)  [unwired: 1 in]
        n361 = Number To Decimal String(number="out") -> (decimal integer string=→"текущая скорость\n(mm/min)":string)  [unwired: 1 in]
        n362 = Number To Fractional String(number="SP_зазор", precision (6)=i16 1) -> (F-format string=→"Задание \nзазора (mm)":string)  [unwired: 2 in]
        n363 = Number To Fractional String(number="V7045_I_ist", precision (6)=i16 0) -> (F-format string=→"I_ist":string)  [unwired: 2 in]
        n364 = Number To Fractional String(number="PV_зазор", precision (6)=i16 1) -> (F-format string=→"текущее значение\nзазора (mm)":string)  [unwired: 2 in]
        n365 = Number To Decimal String(number="V7045_U_ist") -> (decimal integer string=→"U_ist":string)  [unwired: 1 in]
        n366 = Divide(x=w694, y=i16 10) -> (x/y=w692:dbl)
        n367 = Number To Decimal String(number="v4065_cкорость подачи") -> (decimal integer string=→"LONGITUDINAL SPEED":string)  [unwired: 1 in]
        n368 = Number To Decimal String(number=w692) -> (decimal integer string=→"Диаметр заг.":string)  [unwired: 1 in]
        n369 = Number To Decimal String(number="v4066_cкорость подачи плазматрона") -> (decimal integer string=→"PLASMATRON SPEED":string)  [unwired: 1 in]
        n370 = Number To Fractional String(number="V5010_SP_C1", precision (6)=i16 2) -> (F-format string=→"SP Presure C1":string)  [unwired: 2 in]
        n371 = Number To Fractional String(number="V5011_SP_He_PC2", precision (6)=i16 2) -> (F-format string=→"SP Presure He PC2":string)  [unwired: 2 in]
        n372 = Number To Fractional String(number="V5012_SP_He_PC2", precision (6)=i16 2) -> (F-format string=→"SP Presure Ar PC2":string)  [unwired: 2 in]
      }
      event "SP Presure Ar PC2": Mouse Down {
        n373 = event-data() -> ()  [unwired: 1 in, 4 out]
        n374 = local read "SP Presure Ar PC2"() -> (w701:string)
        n375 = call "NUMPAD1_9(ПРОГРАММА)1.vi"("МИНИМАЛЬНОЕ ЗНАЧЕНИЕ"=0.0, "МАКСИМАЛЬНОЕ ЗНАЧЕНИЕ"=9.0, "ДЛИННА СЛОВА"=i8 4, "ТЕКУЩЕЕ ЗНАЧЕНИЕ"=w701) -> ("НОВОЕ ЗНАЧЕНИЕ"=w707:string)  [unwired: 7 in]
        n376 = Fract/Exp String To Number(string=w707) -> (number=w706:dbl)  [unwired: 3 in, 1 out]
        n377 = DataSocket Write(8:errorcluster {"status"=FALSE, "code"=0, "source"=""} ("error in (no error)"), 9:250 ("ms timeout (0)"), 10:w706, 11:"opc://localhost/National Instruments.NIOPCServers/CNL_1.PLC1.PRESURE.V5012_SP_PC2") -> (0:w703:errorcluster)  [unwired: 2 out]
        n378 = Unbundle By Name(w703) -> ()  [unwired: 1 out]
      }
      event "SP Presure C1": Mouse Down {
        n379 = event-data() -> ()  [unwired: 1 in, 4 out]
        n380 = local read "SP Presure C1"() -> (w720:string)
        n381 = call "NUMPAD1_9(ПРОГРАММА)1.vi"("МИНИМАЛЬНОЕ ЗНАЧЕНИЕ"=0.0, "МАКСИМАЛЬНОЕ ЗНАЧЕНИЕ"=0.61, "ДЛИННА СЛОВА"=i8 4, "ТЕКУЩЕЕ ЗНАЧЕНИЕ"=w720) -> ("НОВОЕ ЗНАЧЕНИЕ"=w716:string)  [unwired: 7 in]
        n382 = Fract/Exp String To Number(string=w716) -> (number=w714:dbl)  [unwired: 3 in, 1 out]
        n383 = DataSocket Write(8:errorcluster {"status"=FALSE, "code"=0, "source"=""} ("error in (no error)"), 9:250 ("ms timeout (0)"), 10:w714, 11:"opc://localhost/National Instruments.NIOPCServers/CNL_1.PLC1.PRESURE.V5010_SP_C1") -> (0:w711:errorcluster)  [unwired: 2 out]
        n384 = Unbundle By Name(w711) -> ()  [unwired: 1 out]
      }
      event "SP Presure He PC2": Mouse Down {
        n385 = event-data() -> ()  [unwired: 1 in, 4 out]
        n386 = local read "SP Presure He PC2"() -> (w722:string)
        n387 = call "NUMPAD1_9(ПРОГРАММА)1.vi"("МИНИМАЛЬНОЕ ЗНАЧЕНИЕ"=0.0, "МАКСИМАЛЬНОЕ ЗНАЧЕНИЕ"=9.0, "ДЛИННА СЛОВА"=i8 4, "ТЕКУЩЕЕ ЗНАЧЕНИЕ"=w722) -> ("НОВОЕ ЗНАЧЕНИЕ"=w727:string)  [unwired: 7 in]
        n388 = Fract/Exp String To Number(string=w727) -> (number=w726:dbl)  [unwired: 3 in, 1 out]
        n389 = DataSocket Write(8:errorcluster {"status"=FALSE, "code"=0, "source"=""} ("error in (no error)"), 9:250 ("ms timeout (0)"), 10:w726, 11:"opc://localhost/National Instruments.NIOPCServers/CNL_1.PLC1.PRESURE.V5011_SP_PC2") -> (0:w723:errorcluster)  [unwired: 2 out]
        n390 = Unbundle By Name(w723) -> ()  [unwired: 1 out]
      }
      event "ПЛАЗМАТРОН В ИСХОДНОЕ 2": Value Change {
        w764 = "D:\\img\\"
        w753 = enum32{"File", "Clipboard"}."File" ("Target")
        w754 = enum32{"BMP", "EPS", "EMF", "PICT"}."BMP" ("File Type")
        n391 = event-data() -> ()  [unwired: 1 in, 4 out]
        n392 = Get Date/Time In Seconds() -> (seconds since 1Jan1904=w743:timestamp)
        n393 = Get Date/Time String(seconds (now)=w743) -> ()  [unwired: 2 in, 2 out]
        n394 = Format Date/Time String(time format string (%c)="%H_%M_%S", seconds (now)=w743) -> (date/time string=w739:string)  [unwired: 1 in]
        n395 = Concatenate Strings("VOLTAGE-", w739) -> (w737:string)
        n396 = Concatenate Strings("CURRENT", w739) -> (w735:string)
        n397 = Concatenate Strings("PV-", w739) -> (w741:string)
        n398 = Concatenate Strings("FEED-", w739) -> (w731:string)
        n399 = Concatenate Strings(w764, w735) -> (w761:string)
        n400 = Concatenate Strings(w764, w737) -> (w763:string)
        n401 = Concatenate Strings("PULLEYS", w739) -> (w733:string)
        n402 = Concatenate Strings(w764, w741) -> (w762:string)
        n403 = String To Path(string=w761) -> (path=w757:path)
        n404 = String To Path(string=w763) -> (path=w744:path)
        n405 = Concatenate Strings(w764, w731) -> (w759:string)
        n406 = Concatenate Strings(w764, w733) -> (w760:string)
        n407 = String To Path(string=w762) -> (path=w758:path)
        n408 = String To Path(string=w759) -> (path=w755:path)
        n409 = String To Path(string=w760) -> (path=w756:path)
        n410 = invoke on="Скорость толкателя" class="WFChart (strict)" method="Export Image"("FileType"=w754, "Target"=w753, "Path"=w755) -> (error out=w748:errorcluster)  [unwired: 5 in, 7 out]
        n411 = invoke on="Напряжение" class="WFChart (strict)" method="Export Image"(error in=errorcluster {"status"=FALSE, "code"=0, "source"=""} ("error in (no error)"), "FileType"=w754, "Target"=w753, "Path"=w744, "HideGrid"=FALSE ("Hide Grid"), "Overwrite"=FALSE ("Always Overwrite")) -> (error out=w752:errorcluster)  [unwired: 2 in, 7 out]
        n412 = invoke on="Значение зазора" class="WFChart (strict)" method="Export Image"("FileType"=w754, "Target"=w753, "Path"=w758) -> (error out=w751:errorcluster)  [unwired: 5 in, 7 out]
        n413 = invoke on="Ток" class="WFChart (strict)" method="Export Image"("FileType"=w754, "Target"=w753, "Path"=w757) -> (error out=w750:errorcluster)  [unwired: 5 in, 7 out]
        n414 = invoke on="Частота вращения" class="WFChart (strict)" method="Export Image"("FileType"=w754, "Target"=w753, "Path"=w756) -> (error out=w749:errorcluster)  [unwired: 5 in, 7 out]
        n415 = Unbundle(w751) -> ()  [unwired: 3 out]
        n416 = Unbundle(w750) -> ()  [unwired: 3 out]
        n417 = Unbundle(w752) -> ()  [unwired: 3 out]
        n418 = Unbundle(w748) -> ()  [unwired: 3 out]
        n419 = Unbundle(w749) -> ()  [unwired: 3 out]
      }
      event "Порядковый номер": Mouse Down {
        n420 = event-data() -> ()  [unwired: 1 in, 4 out]
        n421 = local read "Порядковый номер"() -> (w769:string)
        n422 = call "NUMPAD1_9.vi"("МИНИМАЛЬНОЕ ЗНАЧЕНИЕ"=-1.0, "МАКСИМАЛЬНОЕ ЗНАЧЕНИЕ"=100.0, "ДЛИННА СЛОВА"=i8 2, "ТЕКУЩЕЕ ЗНАЧЕНИЕ"=w769) -> ("НОВОЕ ЗНАЧЕНИЕ"=w765:string)  [unwired: 7 in]
        n423 = local write "Порядковый номер"(w765) -> ()
      }
      event "PLASMATRON SPEED": Mouse Down {
        n424 = event-data() -> ()  [unwired: 1 in, 3 out]
        n425 = local read "PLASMATRON SPEED"() -> (w770:string)
        n426 = call "NUMPAD1_9.vi"("МИНИМАЛЬНОЕ ЗНАЧЕНИЕ"=0.0, "МАКСИМАЛЬНОЕ ЗНАЧЕНИЕ"=501.0, "ДЛИННА СЛОВА"=i8 3, "ТЕКУЩЕЕ ЗНАЧЕНИЕ"=w770) -> ("НОВОЕ ЗНАЧЕНИЕ"=w772:string)  [unwired: 7 in]
        n427 = Decimal String To Number(string=w772) -> (number=w775:i32)  [unwired: 2 in, 1 out]
        n428 = DataSocket Write(8:errorcluster {"status"=FALSE, "code"=0, "source"=""} ("error in (no error)"), 9:500 ("ms timeout (0)"), 10:w775, 11:"opc://localhost/National Instruments.NIOPCServers/CNL_1.PLC1.PARAM_RASP.SP_PR_PLAZM") -> (0:w778:errorcluster)  [unwired: 2 out]
        n429 = Unbundle(w778) -> ()  [unwired: 3 out]
      }
      event "LONGITUDINAL SPEED": Mouse Down {
        n430 = event-data() -> ()  [unwired: 1 in, 3 out]
        n431 = local read "LONGITUDINAL SPEED"() -> (w783:string)
        n432 = call "NUMPAD1_9.vi"("МИНИМАЛЬНОЕ ЗНАЧЕНИЕ"=0.0, "МАКСИМАЛЬНОЕ ЗНАЧЕНИЕ"=501.0, "ДЛИННА СЛОВА"=i8 3, "ТЕКУЩЕЕ ЗНАЧЕНИЕ"=w783) -> ("НОВОЕ ЗНАЧЕНИЕ"=w781:string)  [unwired: 7 in]
        n433 = Decimal String To Number(string=w781) -> (number=w785:i32)  [unwired: 2 in, 1 out]
        n434 = DataSocket Write(8:errorcluster {"status"=FALSE, "code"=0, "source"=""} ("error in (no error)"), 9:500 ("ms timeout (0)"), 10:w785, 11:"opc://localhost/National Instruments.NIOPCServers/CNL_1.PLC1.PARAM_RASP.OUT_P_SAG_M") -> (0:w788:errorcluster)  [unwired: 2 out]
        n435 = Unbundle(w788) -> ()  [unwired: 3 out]
      }
      event "Максимальная подача (мм/мин)2": Mouse Down {
        n436 = event-data() -> ()  [unwired: 1 in, 3 out]
        n437 = local read "Максимальная подача (мм/мин)2"() -> (w790:string)
        n438 = call "NUMPAD1_9.vi"("МИНИМАЛЬНОЕ ЗНАЧЕНИЕ"=0.1, "МАКСИМАЛЬНОЕ ЗНАЧЕНИЕ"=101.0, "ДЛИННА СЛОВА"=i8 3, "ТЕКУЩЕЕ ЗНАЧЕНИЕ"=w790) -> ("НОВОЕ ЗНАЧЕНИЕ"=w792:string)  [unwired: 7 in]
        n439 = Decimal String To Number(string=w792) -> (number=w791:i32)  [unwired: 2 in, 1 out]
        n440 = DataSocket Write(8:errorcluster {"status"=FALSE, "code"=0, "source"=""} ("error in (no error)"), 9:500 ("ms timeout (0)"), 10:w791, 11:"opc://localhost/National Instruments.NIOPCServers/CNL_1.PLC1.RID.MAX_OUT") -> (0:w798:errorcluster)  [unwired: 2 out]
        n441 = Unbundle(w798) -> ()  [unwired: 3 out]
      }
      event "Регулятор": Value Change {
        n442 = event-data() -> ()  [unwired: 1 in, 2 out]
        n443 = local read "Boolean"() -> (w801:bool)
        n444 = Not(x=w801) -> (.not. x?=w800:bool)
        n445 = DataSocket Write(8:errorcluster {"status"=FALSE, "code"=0, "source"=""} ("error in (no error)"), 9:500 ("ms timeout (0)"), 10:w800, 11:"opc://localhost/National Instruments.NIOPCServers/CNL_1.PLC1.RID.RID_RUN") -> (0:w804:errorcluster)  [unwired: 2 out]
        n446 = Unbundle(w804) -> ()  [unwired: 3 out]
      }
      event "взять зазор": Value Change {
        n447 = event-data() -> ()  [unwired: 1 in, 3 out]
        n448 = DataSocket Write(8:errorcluster {"status"=FALSE, "code"=0, "source"=""} ("error in (no error)"), 9:500 ("ms timeout (0)"), 10:TRUE, 11:"opc://localhost/National Instruments.NIOPCServers/CNL_1.PLC1.RID.PV_to_SP") -> (0:w808:errorcluster)  [unwired: 2 out]
        n449 = Unbundle(w808) -> ()  [unwired: 3 out]
      }
      event "Задание \nзазора (mm)": Mouse Down {
        n450 = event-data() -> ()  [unwired: 1 in, 2 out]
        n451 = local read "Задание \nзазора (mm)"() -> (w813:string)
        n452 = call "NUMPAD1_9(ПРОГРАММА).vi"("МИНИМАЛЬНОЕ ЗНАЧЕНИЕ"=0.09, "МАКСИМАЛЬНОЕ ЗНАЧЕНИЕ"=100.0, "ДЛИННА СЛОВА"=i8 4, "ТЕКУЩЕЕ ЗНАЧЕНИЕ"=w813) -> ("НОВОЕ ЗНАЧЕНИЕ"=w814:string)  [unwired: 7 in]
        n453 = Fract/Exp String To Number(string=w814) -> (number=w811:dbl)  [unwired: 3 in, 1 out]
        n454 = DataSocket Write(8:errorcluster {"status"=FALSE, "code"=0, "source"=""} ("error in (no error)"), 9:500 ("ms timeout (0)"), 10:w811, 11:"opc://localhost/National Instruments.NIOPCServers/CNL_1.PLC1.RID.SP_ZAZOR") -> (0:w819:errorcluster)  [unwired: 2 out]
        n455 = Unbundle(w819) -> ()  [unwired: 3 out]
      }
      event "Марка сплава": Mouse Down {
        n456 = event-data() -> ()  [unwired: 1 in, 4 out]
        n457 = local read "Марка сплава"() -> (w821:string)
        n458 = call "КЛАВИАТУРА ПОЛНАЯSMALL.vi"("ВХОД СТАРОЕ"=w821) -> ("ВЫХОД РЕЗУЛЬТАТ"=→"Марка сплава":string)  [unwired: 10 in]
      }
      event "откачка стоп 2": Value Change {
        n459 = event-data() -> ()  [unwired: 1 in, 4 out]
        n460 = call "8.1 форма проверки натекания.vi"() -> ()  [unwired: 1 in]
      }
    }
  }
  n461 = while {
    stop <- "stop 3" stop-if-true
    n462 = Wait (ms)(milliseconds to wait=u32 100) -> ()  [unwired: 1 out]
    n463 = local read "16bit integer"() -> (w824:i16)
    n464 = DataSocket Write(8:errorcluster {"status"=FALSE, "code"=0, "source"=""} ("error in (no error)"), 9:100 ("ms timeout (0)"), 10:w824, 11:"opc://localhost/National Instruments.NIOPCServers/CNL_1.PLC1.RID.PV_ZAZOR") -> (0:w825:errorcluster)  [unwired: 2 out]
    n465 = Unbundle(w825) -> ()  [unwired: 3 out]
  }
  n466 = while {
    stop <- FALSE stop-if-true
    n467 = flat-sequence {
      tunnel: [w845] -> w838
      tunnel: [w844] -> w832
      tunnel: [w843] -> w830
      tunnel: w838 -> [w856]
      tunnel: [w855] -> w837
      tunnel: [w850] -> w833
      tunnel: w832 -> [w850]
      tunnel: w830 -> [w848]
      tunnel: w837 -> [w864]
      tunnel: [w863] -> w835
      tunnel: [w862] -> w834
      tunnel: w833 -> [w862]
      tunnel: w835 -> [_]
      tunnel: w834 -> [_]
      frame #0 {
        "Запись" <- FALSE ("Rec.")
      }
      frame #1 {
        n468 = while {
          stop <- "Запись отчета" stop-if-true
          n469 = Wait Until Next ms Multiple(millisecond multiple=u32 1000) -> ()  [unwired: 1 out]
        }
      }
      frame #2 {
        n470 = local read "Порядковый номер"() -> (w843:string)
        n471 = local write "Запись"(TRUE ("Rec.")) -> ()
        n472 = call "1.1.путь каталога отчета цикла.vi"("bilet_numer"=w843) -> ("path_out"=w844:string)  [unwired: 10 in]
        n473 = Concatenate Strings(w844, "rasp.txt" ("string")) -> (w846:string)
        n474 = String To Path(string=w846) -> (path=w845:path)
      }
      frame #3 {
        n475 = local read "Марка сплава"() -> (w849:string)
        n476 = Get Date/Time In Seconds() -> (seconds since 1Jan1904=w852:timestamp)
        n477 = Format Date/Time String(seconds (now)=w852) -> (date/time string=w851:string)  [unwired: 2 in]
        n478 = Concatenate Strings(w851, "  WORK ", w849, " NUMBER - ", w848) -> ()  [unwired: 1 out]
        n479 = Open/Create/Replace File(file path (use dialog)=w856, error in=errorcluster {"status"=FALSE, "code"=0, "source"=""}, operation (0:open)=T6."open or create") -> (refnum out=w861:refnum<file>, error out=w860:errorcluster)  [unwired: 3 in, 1 out]
        n480 = Close File(refnum=w861, error in=w860) -> (path=w855:path, error out=w859:errorcluster)
        n481 = Unbundle(w859) -> ()  [unwired: 3 out]
        "Порядковый номер" <- w848
      }
      frame #4 {
        n482 = while {
          tunnel: w864 -> [w882]
          tunnel: [w876] -> w863
          stop <- w892 stop-if-true
          w879 = "\t"
          n483 = local read "Запись отчета"() -> (w875:bool)
          n484 = Wait Until Next ms Multiple(millisecond multiple=u32 1000) -> ()  [unwired: 1 out]
          n485 = local read "текущая скорость\n(mm/min)"() -> (w871:string)
          n486 = local read "Порядковый номер"() -> (w877:string)
          n487 = local read "P плазматрон (bar)"() -> (w866:string)
          n488 = local read "V вращ. бараб"() -> (w872:string)
          n489 = local read "Марка сплава"() -> (w865:string)
          n490 = Get Date/Time In Seconds() -> (seconds since 1Jan1904=w874:timestamp)
          n491 = local read "Диаметр заг."() -> (w873:string)
          n492 = local read "P камера (bar)"() -> (w867:string)
          n493 = Format Date/Time String(seconds (now)=w874) -> (date/time string=w880:string)  [unwired: 2 in]
          n494 = Not(x=w875) -> (.not. x?=w892:bool)
          n495 = local read "текущее значение\nзазора (mm)"() -> (w868:string)
          n496 = local read "U_ist"() -> (w869:string)
          n497 = Open/Create/Replace File(file path (use dialog)=w882, error in=errorcluster {"status"=FALSE, "code"=0, "source"=""}) -> (refnum out=w891:refnum<file>, error out=w889:errorcluster)  [unwired: 4 in, 1 out]
          n498 = local read "I_ist"() -> (w870:string)
          n499 = Concatenate Strings(w880, w879, w873, w879, w872, w879, w871, w879, w870, w879, w869, w879, w868, w879, w867, w879, w866, w879, w865, w879, w877, "\r") -> (w881:string)
          n500 = Set File Position(refnum=w891, from (0:start)=enum16{"start", "end", "current"}."end", error in=w889) -> (refnum out=w888:refnum<file>, error out=w887:errorcluster)  [unwired: 1 in]
          n501 = Write to Text File(file (use dialog)=w888, text=w881, error in=w887) -> (refnum out=w886:refnum<file>, error out=w885:errorcluster)  [unwired: 1 in, 1 out]
          n502 = Close File(refnum=w886, error in=w885) -> (path=w876:path, error out=w884:errorcluster)
          n503 = Unbundle(w884) -> ()  [unwired: 3 out]
        }
      }
      frame #5 {
      }
    }
    n504 = Wait Until Next ms Multiple(millisecond multiple=u32 1000) -> ()  [unwired: 1 out]
  }
  n505 = local write "Порядковый номер"("0" ("Порядковый номер")) -> ()
  n506 = while {
    stop <- FALSE stop-if-true
    n507 = flat-sequence {
      tunnel: [w989] -> w896
      frame #0 {
        n508 = call <vilib>:"Application Directory.vi"() -> ("Application Directory"=w903:path)
        n509 = Path To String(path=w903) -> (string=w902:string)
        n510 = Concatenate Strings(w902, "\\set_cam" ("string")) -> (w900:string)
        n511 = String To Path(string=w900) -> (path=w897:path)
        n512 = Get File Size(file=w897) -> (0:w899:errorcluster)  [unwired: 1 in, 2 out]
        n513 = Unbundle By Name(w899) -> ("status"=w898:bool)
        n514 = case shown="False" w898 {
          tunnel: w897 -> [w976 _]
          frame False {
            n515 = call-poly <vilib>:"Read From Spreadsheet File.vi"("file path (dialog if empty)"=w976) -> ("first row"=w975:string[])  [unwired: 6 in, 4 out]
            n516 = Index Array(array=w975, index #1=0 ("index"), index #2=2 ("index"), index #3=3 ("index"), index #4=4 ("index"), index #5=5 ("index"), index #6=6 ("index"), index #7=7 ("index"), index #8=8 ("index"), index #9=9 ("index"), index #10=10 ("index"), index #11=11 ("index"), index #12=12 ("index"), index #13=13 ("index"), index #14=14 ("index"), index #15=15 ("index"), index #16=16 ("index"), index #17=17 ("index"), index #18=18 ("index"), index #19=19 ("index"), index #20=20 ("index"), index #21=21 ("index")) -> (element #1=w973:string, element #2=w971:string, element #3=w968:string, element #4=w960:string, element #5=w958:string, element #6=w956:string, element #7=w954:string, element #8=w952:string, element #9=w943:string, element #10=w941:string, element #11=w939:string, element #12=w937:string, element #13=w935:string, element #14=w933:string, element #15=w931:string, element #16=w929:string, element #17=w919:string, element #18=w914:string, element #19=w912:string, element #20=w908:string, element #21=w904:string)
            n517 = local write "Камера"(w973) -> ()
            n518 = Decimal String To Number(string=w971) -> (number=w970:i32)  [unwired: 2 in, 1 out]
            n519 = Decimal String To Number(string=w960) -> (number=w965:i32)  [unwired: 2 in, 1 out]
            n520 = Decimal String To Number(string=w958) -> (number=w964:i32)  [unwired: 2 in, 1 out]
            n521 = Decimal String To Number(string=w956) -> (number=w963:i32)  [unwired: 2 in, 1 out]
            n522 = Decimal String To Number(string=w954) -> (number=w962:i32)  [unwired: 2 in, 1 out]
            n523 = Fract/Exp String To Number(string=w952) -> (number=w951:dbl)  [unwired: 3 in, 1 out]
            n524 = Decimal String To Number(string=w968) -> (number=w967:i32)  [unwired: 2 in, 1 out]
            n525 = Decimal String To Number(string=w943) -> (number=w949:i32)  [unwired: 2 in, 1 out]
            n526 = Decimal String To Number(string=w941) -> (number=w948:i32)  [unwired: 2 in, 1 out]
            n527 = Decimal String To Number(string=w939) -> (number=w947:i32)  [unwired: 2 in, 1 out]
            n528 = Decimal String To Number(string=w937) -> (number=w946:i32)  [unwired: 2 in, 1 out]
            n529 = Decimal String To Number(string=w935) -> (number=w928:i32)  [unwired: 2 in, 1 out]
            n530 = Decimal String To Number(string=w933) -> (number=w926:i32)  [unwired: 2 in, 1 out]
            n531 = Decimal String To Number(string=w931) -> (number=w924:i32)  [unwired: 2 in, 1 out]
            n532 = Decimal String To Number(string=w929) -> (number=w922:i32)  [unwired: 2 in, 1 out]
            n533 = Decimal String To Number(string=w919) -> (number=w918:i32)  [unwired: 2 in, 1 out]
            n534 = Decimal String To Number(string=w914) -> (number=w913:i32)  [unwired: 2 in, 1 out]
            n535 = Decimal String To Number(string=w912) -> (number=w911:i32)  [unwired: 2 in, 1 out]
            n536 = Decimal String To Number(string=w908) -> (number=w910:i32)  [unwired: 2 in, 1 out]
            n537 = Decimal String To Number(string=w904) -> (number=w906:i32)  [unwired: 2 in, 1 out]
            n538 = local write "Задержка"(w970) -> ()
            n539 = local write "Фильтр"(w967) -> ()
            n540 = local write "Рабочий цвет"(w906) -> ()
            n541 = local write "Калибровка"(w918) -> ()
            n542 = Bundle(w965, w964, w963, w962, w951) -> (w966:cluster{i32, i32, i32, i32, dbl})  [unwired: 1 in]
            n543 = To Unsigned Long Integer(number=w946) -> (unsigned 32bit integer=w945:u32)
            n544 = call "конвертюга.vi"("Numeric"=w928) -> ("Boolean"=w927:bool)  [unwired: 10 in]
            n545 = call "конвертюга.vi"("Numeric"=w926) -> ("Boolean"=w925:bool)  [unwired: 10 in]
            n546 = call "конвертюга.vi"("Numeric"=w924) -> ("Boolean"=w923:bool)  [unwired: 10 in]
            n547 = call "конвертюга.vi"("Numeric"=w922) -> ("Boolean"=w921:bool)  [unwired: 10 in]
            n548 = call "конвертюга.vi"("Numeric"=w910) -> ("Boolean"=w909:bool)  [unwired: 10 in]
            n549 = Bundle(w913, w911) -> (w917:cluster{i32, i32})  [unwired: 1 in]
            n550 = local write "Область измерения"(w966) -> ()
            n551 = local write "Уровень бинаризации"(w917) -> ()
            n552 = local write "Blank Button"(w909) -> ()
            n553 = Bundle(w949, w948, w947, w945, "Boolean"=w927, "Boolean"=w925, "Boolean"=w923, "Boolean"=w921) -> (w950:T8)  [unwired: 1 in]
            n554 = local write "Параметры измерения"(w950) -> ()
          }
          frame True {
          }
        }
      }
      frame #1 {
        n555 = case shown="True" FALSE {
          frame False {
          }
          frame True {
            n556 = while {
              stop <- "Play Button" stop-if-true
              "Индикатор камеры" <- FALSE ("Индикатор камеры")
            }
          }
        }
      }
      frame #2 {
        w981 = T9 4 items=["Grayscale (U8)", "Grayscale (I16)", "Grayscale (SGL)", "Complex (CSG)", "RGB (U32)", "HSL (U32)", "RGB (U64)", "Grayscale (U16)"] ("Image Type")
        w986 = T9 4 items=["Grayscale (U8)", "Grayscale (I16)", "Grayscale (SGL)", "Complex (CSG)", "RGB (U32)", "HSL (U32)", "RGB (U64)", "Grayscale (U16)"] ("Image Type")
        n557 = call <vilib>:"IMAQdx Open Camera.vi"("Session In"="Камера") -> ("Session Out"=w988:T10)  [unwired: 9 in, 1 out]
        n558 = call <vilib>:"IMAQdx Configure Grab.vi"("Session In"=w988) -> ("Session Out"=w984:T10)  [unwired: 9 in, 1 out]
        n559 = call "IMAQ Create"("Image Name"="capture", "Image Type"=w986) -> ("New Image"=w983:T5)  [unwired: 3 in, 1 out]
        n560 = call "IMAQ Create"("Image Name"="capture2", "Image Type"=w981) -> ("New Image"=w980:T5)  [unwired: 3 in, 1 out]
        n561 = while {
          tunnel: [w1003] -> w989
          tunnel: w984 -> [w993]
          tunnel: w983 -> [w992]
          tunnel: w980 -> [w990]
          stop <- "Media Stop Button" stop-if-true
          n562 = flat-sequence {
            tunnel: [w1007] -> w1002
            tunnel: [w1004] -> w1000
            tunnel: w993 -> [w1006]
            tunnel: w992 -> [w1005]
            tunnel: [w1004] -> w991
            tunnel: w1002 -> [w1018]
            tunnel: [w1018] -> w1001
            tunnel: w1000 -> [w1017]
            tunnel: [w1017] -> w999
            tunnel: w991 -> [w1016]
            tunnel: w990 -> [w1012]
            tunnel: w1001 -> [w1038]
            tunnel: w999 -> [w1037]
            tunnel: [w1038] -> w998
            tunnel: [w1036] -> w995
            tunnel: w998 -> [w1060]
            tunnel: [w1060] -> w997
            tunnel: [w1059] -> w996
            tunnel: w995 -> [w1059]
            tunnel: [w1062] -> w1003
            tunnel: w997 -> [w1062]
            tunnel: w996 -> [w1061]
            frame #0 {
              n563 = local write "Индикатор камеры"(TRUE ("Индикатор камеры")) -> ()
              n564 = call <vilib>:"IMAQdx Grab.vi"("Image In"=w1005, "Session In"=w1006) -> ("Image Out"=w1004:T5, "Session Out"=w1007:T10)  [unwired: 6 in, 2 out]
            }
            frame #1 {
              w1011 = u32 1 items=["Horizontal", "Vertical", "Central", "1st Diagonal", "2nd Diagonal"] ("Type of Symmetry")
              n565 = call "IMAQ Copy"("Image Dst"=w1012, "Image Src"=w1016) -> ("Image Dst Out"=w1014:T5)  [unwired: 4 in, 1 out]
              n566 = call "IMAQ Symmetry"("Type of Symmetry"=w1011, "Image Dst"=w1012, "Image Src"=w1014) -> ("Image Dst Out"=w1013:T5)  [unwired: 2 in, 1 out]
              n567 = call-poly "IMAQ Write File 2"("error in (no error)"=errorcluster {"status"=FALSE, "code"=0, "source"=""}, "File Path"=path "D:/image", "Image"=w1013) -> ("error out"=w1009:errorcluster)  [unwired: 7 in, 1 out]
              n568 = Unbundle(w1009) -> ()  [unwired: 3 out]
            }
            frame #2 {
              (unwired) 7 items=["Red", "Green", "Blue", "Hue", "Saturation", "Luminance", "Value", "Intensity"] ("Color Plane")
              (unwired) u32 8487297 ("Color Box")
              (unwired) 612
              n569 = Wait (ms)(milliseconds to wait="Задержка") -> ()  [unwired: 1 out]
              n570 = Increment(x="Numeric") -> (x+1=w1039:i16)
              n571 = local write "Numeric"(w1039) -> ()
              n572 = call "IMAQ Subtract"("Image Src A"=w1037, "Constant"="Калибровка") -> ("Image Dst Out"=w1047:T5)  [unwired: 5 in, 1 out]
              n573 = call "IMAQ ExtractSingleColorPlane"("Color Plane"="Фильтр", "Image Src"=w1047) -> ("Image Dst Out"=w1026:T5)  [unwired: 8 in, 1 out]
              n574 = Unbundle("Область измерения") -> ("Top"=w1023:i32, "Bottom"=w1022:i32)  [unwired: 3 out]
              n575 = Greater?(x=w1023, y=w1022) -> (0:w1025:bool)
              n576 = case shown="True" "Blank Button" {
                tunnel: w1026 -> [w1054 w1058]
                tunnel: [w1054 w1057] -> w1033
                frame False {
                }
                frame True {
                  (unwired) cluster{"Lower value":sgl, "Upper value":sgl} {"Lower value"=124.0, "Upper value"=255.0} ("Range")
                  (unwired) u32 16448250 ("Color Box 2")
                  n577 = call "IMAQ Threshold"("Replace Value"="Рабочий цвет", "Range"="Уровень бинаризации", "Image Src"=w1058) -> ("Image Dst Out"=w1057:T5)  [unwired: 3 in, 5 out]
                }
              }
              n578 = case shown="False" w1025 {
                tunnel: [w1051 w1053] -> w1024
                tunnel: w1023 -> [w1050 w1053]
                tunnel: w1022 -> [w1051 w1052]
                tunnel: [w1050 w1052] -> w1021
                frame False {
                }
                frame True {
                }
              }
              n579 = Subtract(x=w1024, y=w1021) -> (x-y=w1031:i32)
              n580 = Multiply(x="D, заготовки", y=i16 10) -> (x*y=w1028:i16)
              n581 = Divide(x=w1028, y=w1031) -> (x/y=w1027:dbl)
              "x/y" <- w1027
              n582 = call "IMAQ Clamp Horizontal Max"("Settings"="Параметры измерения", "Rectangle"="Область измерения", "Image"=w1033) -> ("Distance"=w1045:sgl, "Image Out"=w1036:T5)  [unwired: 4 in, 3 out]
              "Distance зазор" <- w1045
              n583 = Multiply(x=w1045, y=w1027) -> (x*y=w1043:dbl)
              "x*y" <- w1043
              n584 = Divide(x=w1043, y=10.0) -> (x/y=w1041:dbl)
              n585 = Divide(x=800, y=574) -> ()  [unwired: 1 out]
              n586 = To Word Integer(number=w1041) -> (16bit integer=→"16bit integer":i16)
              "Индикатор камеры 2" <- "Blank Button"
            }
            frame #3 {
            }
            frame #4 {
              "индикация видео" <- w1061
            }
          }
        }
      }
    }
    n587 = Wait Until Next ms Multiple(millisecond multiple=u32 10) -> ()  [unwired: 1 out]
    n588 = call <vilib>:"IMAQdx Close Camera.vi"("Session In"=w896) -> ()  [unwired: 10 in, 1 out]
  }
